vi "Phoenix.vi"(9 "Com UDP":T13={"UDP GrSim TX"=TRUE, "Address:"="", "Port:"=20011}, 10 "RefBox UDP RX":T12={"Local IP:"="192.168.2.61", "Server IP:"="224.5.23.1", "Port"="10003"}, 11 "SSL UDP RX":T12={"Local IP:"="", "Server IP:"="224.5.23.2", "Port"="10020"}) -> ()   [LabVIEW 2024]
uses:
  Vision_class/Old vision/Controls/Estimadores.ctl
  Vision_class/Old vision/Decode SSL and Refree Wrapper Package Folder/SSL Referee Game Status.ctl
  Vision_class/Old vision/Draw Field Folder/DrawTargets.ctl
  Vision_class/Old vision/Controls/SSL Field State.ctl
  Vision_class/Old vision/Controls/SSL Detection Frame.ctl
  Vision_class/Old vision/Controls/SSL Detection Robot.ctl
  <vilib>/Analysis/Matrix/Datatypes/RealMatrix.ctl
  Vision_class/Old vision/Controls/SSL Detection Ball.ctl
  Communication_class/Communication.lvclass
  Controls/ComUDP.ctl
  Controls/ComSerial.ctl
  Controls/ComSOS.ctl
  Controls/PhoenixParameters.ctl
  Play_class/PassReceiver.ctl
  Parameters_class/ChoosePassReceiver.ctl
  Game_class/Navigation/Controls/bangBangControlParameters.ctl
  Game_class/PathPlanning/Path Planning/RRT/RRTParameters.ctl
  Controls/PIDParameters.ctl
  Parameters_class/Project.ctl
  Controls/RobotModelTestState.ctl
  Game_class/VelocityPlanningTest/Controls/testMode.ctl
  Controls/RobotModelReplacementTest.ctl
  Controls/grSimReplacement.ctl
  Communication_class/Paths/grSim Packet Command UDP Test Folder/grSim/grSim RobotReplacement.ctl
  Communication_class/Paths/grSim Packet Command UDP Test Folder/grSim/grSim_BallReplacement.ctl
  Game_class/KickValueTest/KickValuetest.ctl
  Game_class/KickValueTest/KickValue.ctl
  Game_class/KickValueTest/BallValue.ctl
  Game_class/VelocityPlanningTest/Controls/velocityPlanningState.ctl
  Game_class/VelocityPlanningTest/Controls/trajectoryState.ctl
  Controls/Enviroment.ctl
  Team_class/KeeperPlay.ctl
  Team_class/OffensivePlay.ctl
  Referee_class/command_interpreted.ctl
  Robot_class/roles.ctl
  Robot_class/tactics.ctl
  Team_class/DefensivePlay.ctl
  Controls/vision_control.ctl
  Game_class/KickForceTest/Controls/kickForceTestState.ctl
  Game_class/KickForceTest/Controls/KickForceEnum.ctl
  Game_class/Replay/ReplayControls.ctl
  Game_class/ParametersFromFile/ParametersFromFile.ctl
  Robot_class/robotDisplayFeedback.ctl
  Controls/NewParameters.ctl
  Utilities_class/Style.ctl
  Controls/AllyTeam.ctl
  Zone_class/zones.ctl
  Vision_class/Vision.lvclass
  Game_class/Game.lvclass
  Vision_class/Old vision/Controls/SSL_BallModelStraightTwoPhase.ctl
  Game_class/Game.lvclass/Game.ctl
  Referee_class/Referee.lvclass/Referee.ctl
  Team_class/Team.lvclass/Team.ctl
  Robot_class/Robot.lvclass/Robot.ctl
  Game_class/ParametersFromFile/MainGameConfigs.ctl
  Robot_class/Robot.lvclass
  Events_class/Events.lvclass
  RobotFeedback/RobotFeedback.lvclass/RobotFeedback.ctl
  RobotFeedback/Read id.vi
  RobotFeedback/Read dribblerContactToBall.vi
  Game_class/Write RobotsFeedback.vi
  Robot_class/Read id.vi
  Robot_class/Read role.vi
  Robot_class/Read tactic.vi
  Game_class/Read Referee.vi
  Game_class/Read KeeperTeam.vi
  Game_class/Read OffensiveTeam.vi
  Game_class/Read DefensiveTeam.vi
  Team_class/Read RobotRef.vi
  Team_class/Read DefensivePlay.vi
  Team_class/Read OffensivePlay.vi
  Team_class/Read KeeperPlay.vi
  Referee_class/Read command_interpreted.vi
  Game_class/Write TestTeam.vi
  Game_class/Write DefensiveTeam.vi
  Game_class/Read AllyRef.vi
  Team_class/Write RobotRef.vi
  Game_class/Write NavigationTeam.vi
  Game_class/Write EventsRef.vi
  Game_class/Write OffensiveTeam.vi
  Game_class/Write KeeperTeam.vi
  Ally_class/Ally.lvclass
  C:/Users/moise/Documents/GitHub/SSL_AI/Team_class/Team.lvclass
  RobotFeedback/commCAS.vi
  Referee_class/Referee.lvclass
  Playbook_class/Playbook.lvclass
  <vilib>/Analysis/Matrix/NI_Matrix.lvlib
  Utilities_class/Utilities.lvclass
  RobotFeedback/RobotFeedback.lvclass
  Zone_class/Zone.lvclass
panel:
  in  "accel":dbl
  out "topSpeed":dbl=2466.234375
  out "FPS vision":dbl=64.30864933106373
  out "kick":bool
  in  "Enum":T1=enum."Size"
  in  "Boolean":bool
  in  "robotAngles":dbl[](array[numeric])=[30.0, 150.0, 225.0, 315.0] format="%#_13g"
  out "LastOffensivePlays":T2[](array[typedef])=[enum."5RobotsNormalGamePlay", enum."EnemyPossesionAtOurField", enum."5RobotsNormalGamePlay"]
  out "FPS Read UPD by Cam":dbl=235.84891019160068
  out "DefenseAvoidArea":bool
  in  "AttackerAvoidArea":bool
  out "KeeperPlay":T3=enum."KeeperPlay"
  out "OffensivePlay":T2=enum."5RobotsNormalGamePlay"
  out "DefensivePlay":T4=enum."NormalDefensive"
  out "command_interpreted":T5=enum."Force Start"
  out "robotFeedback":cluster{"id":u32, "dribblerContact":bool}[](array[cluster])
  in  "Life Time":dbl=2.5
  in  "timeToValidateBall":dbl=1.0
  in  "Line?":bool
  in  "BallOut":bool
  out "replaceBall":bool
  out "replaceRobots":bool
  out "grSIM replacement":T6
  out "robotControlResponseConnectionID":refnum<k16>
  out "robotControlResponseErrorOut":errorcluster
  out "error out 2":errorcluster={"status"=TRUE, "code"=66, "source"="UDP Read in Phoenix.vi"}
  in  "Debug Ball":bool
  out "NaN?":bool
  out "Log":string
  out "Exit":i32
  in  "Args":string[](array[string])
  out "touch":bool
  in  "Field Size":T9
  in  "Debug":bool=TRUE
  in  "ball velocity máx":dbl=8.0
  in  "ChipKick activated":bool=TRUE
  out "error out":errorcluster
  in  "Draw Graphs":bool
  in  "Test":bool
  in  "Tab Control":T10(tab)=enum."NewParameters"
  in  "ParametersFromFile":T11
  in  "Com Serial":T14={"Serial TX"=TRUE, "Porta:"="COM4"}
  in  "Com SOS":T15={"UDP SOS TX "=FALSE, "SOS Port: 2"=10025, "SOS Port: "=10021, "SOS Address:"="192.168.0.101"}
  out "RefBox RX":bool=TRUE
  in  "Defense\n stretch":i32=2000
  in  "Defense\n width":i32=1000
  in  "Team":enum16{"Azul", "Amarelo"}(ring) caption="Enum"
  in  "Side":enum16{"Esquerdo", "Direito"}(ring) caption="Enum"
  in  "Command":string(combo)="Force Start"
  in  "AttakingOurselves":bool
  out "SSL RX":bool=TRUE
  in  "FIRASim?":bool
  in  "Project":T16
  in  "Envirnoment":T17=enum."realGame"
  in  "ViewState":T18(ring)=enum."Maximized"
  out "RefBox RX 2":bool=TRUE
  out "SSL RX":bool=TRUE
  out "displayFeedbackRobot":T19[](array[typedef]) {"Battery (V)" scale=6.0..8.4}
  out "Side out":enum16{"Esquerdo", "Direito"}(ring) caption="Enum"
  out "Team out":enum16{"Azul", "Amarelo"}(ring) caption="Enum"
  out "Envirnoment out":T17=enum."realGame"
  in  "AI Parameters":T20={"Defensive Marker"=enum."SecondMostDangerous", "TimeoutDistanceInX"=600.0, "TimeoutDistanceInY"=600.0, "DistanceForaStillBall"=0.0, "TouchDistance"=150.0, "AttackerFarback"=1500.0, "MinDistToKick"=400.0, "Type of Marker"=enum."BlockOurGoal", "Type of Defense "=enum."Barreira", "PassAngle"=0.045, "KickRange"=60.0, "KickForce"=34.0, "KickEps"=0.1, "KickAngle"=5.0, "PassForceMult"=1.2, "DistanceToKickingAngle"=150.0, "DistanceToBallOut"=600.0, "DistanceStop"=750.0, "DistanceBehindAttacker"=200.0, "Area"=enum."Square", "DistanceForPossession"=350.0, "DistanceToConsirerRobotArrive"=50.0, "DistanceToGoAroundBall"=60.0, "DistanceInFrontOfAttacker"=200.0, "TimeoutDistanceBetweenRobots"=300.0, "MaxOutputAngle"=3.0, "MaxOutputXY"=3.5, "MaxDeceleration"=1.0, "MaxControlIncrement"=1.0, "MaxAcceleration"=4.5, "AngularToleranceForPossession"=0.3, "MaxVelBallToBeginDuelist"=0.5, "ZigZagAngle"=0.0, "PID gains Vel"={"(Kc)"=0.1, "(Ti, min)"=0.0, "(Td, min)"=2.0}, "Number of Offensive"=enum."Auto", "Shoot Out?"=FALSE, "DefenseAvoidArea"=FALSE, "InvertKick"=[], "Simple Pass"=FALSE, "ShootOutForce"=20.0, "dtPosEstBall"=0.3, "AttkIgnoreBallObst"=2500.0, "BarrierDist"=130.0, "PassReceiver"=enum."Auto", "GoalieInFrontGoal"=120.0, "RollToPass"=FALSE, "PassReceiver"=enum."Auto", "OldRRT"=FALSE, "Dribbler"=FALSE, "VelNearBall"=2.0, "ChipKick Force"=2.5, "ForcePass\nInGame"=10.0, "bangBangParameters"={"MaxVSent"=4.0, "MaxVNorm"=4.0, "MaxVAng"=8.0, "VAngCircle"=3.0, "LBeginCircle"=300.0, "DistToDestOrientation"=300.0, "MaxVAngToTurn"=8.0, "AtkDistToDestOrientation"=3500.0, "KepperMaxVSent"=4.0, "VelNearEnemy"=1.5}, "BallVelToAbortPass"=0.1, "BallVelToFinishPass"=1.0, "minDistanceToPass"=1000.0, "dribbler_rpm"=1.0, "AttackerAngle\nToTurnInDegrees"=5.0, "AttackerAngle\nToShootInDegrees"=0.5, "distToActivateDibbler"=1000.0, "StopVelocity"=1.2, "timeoutToShoot"=10.0, "DistanceArea"=100.0, "MinDistanceEnemy\nToBallToMark"=750.0, "DisableStopAvoidArea"=FALSE, "RRT Parameters"={"threshold"=120.0, "Step"=120.0, "GoalProb"=0.1, "WayPointProb"=0.6}, "PID per ID"=[]} {"RRT Parameters"."WayPointProb" format="%#_13g"; "RRT Parameters"."GoalProb" format="%#_13g"}
  in  "NewParameters":T26={"PenaltyDistance"=1800.0, "DistanceAttackerToBackBall"=40.0, "Division"=enum."Div B", "DistanceToAvoidyEnemyRobot"=600.0, "BallPlacementDistance"=900.0, "DisatanceBehindBallToStealBall"=600.0, "MaxDistanceToPositionKickoff"=2000.0, "BlockEnemyTarget"=TRUE, "MaxStopVAng"=4.0, "DistanceMarkerToEnemy"=600.0, "IgnoreDribblerContact"=FALSE, "DistanceToBeginEnemyPosession"=400.0, "GoToBallWhenEnemyNotMoving"=TRUE, "EnemyDistanceToReduceVelocity"=500.0, "TurnOnEnemyDistanceToReduceVelocity"=TRUE, "EnemyDistanceToShootOutBall"=0.0, "DefenseKickBall"=TRUE, "MoreKickToGoal? (0-0.3)"=0.25, "ChipKickInEnemyField"=TRUE, "ShootOutRobotId"=4.0, "FieldLenghtDenominatorInShootOut"=-18.0, "AdjustPositionInBallPlacement"=FALSE, "PowerGodPass"=0.75, "VelocityAbortEnemyPos"=3.0, "MaxDistToBeginPass"=300.0, "MinDistToBeginPass"=150.0, "VelocityInDirects"=0.3, "BadDribblerIDs"=[], "NewKickToDistanceAroundBall"=300.0, "PowerAvoidColisionMarker"=1.0, "DistanceToAvoidColisionMarker"=0.0, "AvoidBallKick"=70.0, "DistanceTryKick"=-250.0, "SuicideKickDIstance"=80.0, "AdjustFirstKickDistance"=100.0, "AvoidAimLessKick"=0.7, "DistanceToAvoidyEnemyShootRobot "=100.0, "NumberOfMarkers"=1.0, "PotField"=FALSE, "PIDLateral"=TRUE, "MinDistanceFirstKickX"=100.0, "MinDistanceFirstKickY"=750.0, "FractionOfDistToTouchGround\nAfterChipKick"=0.7, "FractionOfKickxWhen\nComposedWithKickz"=0.7, "Style"=enum."Offensive", "MoveInTurnState"=TRUE, "DistFromEnemyToConsider\nMoveInTurnState"=400.0, "CascadePID"=TRUE, "TurnAroundParameters"={"Radius"=270.0, "Multiplier"=2.0, "ChordAngle"=100.0}, "SafeDriveVel"=0.2, "DistanceToGoToBackBall"=500.0, "minDistanceToNotFinish\nEnemyPossession"=100.0, "OneTouchShot"={"angleFactor"=1.0, "maxAngle"=70.0, "Attack"=TRUE, "Defense"=TRUE}, "OpenAngleToGoal"={"minAngle"=2.0, "maxAngle"=15.0, "minEvaluation"=0.5}, "ShotInterception"={"shotSpeed"=6.0, "minEnemySpeed"=0.7, "maxEnemySpeed"=2.5, "minEvaluation"=0.5}, "AllyTeamArray"=[enum."Defender", enum."Defender", enum."Keeper", enum."Attacker", enum."Attacker", enum."Attacker"], "maxDefendersNumber"=2, "Zone"={"GuardPositionArray"=[[1000.0, 0.0], [1000.0, 1500.0], [1000.0, -1500.0], [875.0, 0.0], [3125.0, 1750.0], [3125.0, -1750.0], [875.0, 1500.0], [875.0, -1500.0], [3125.0, 1750.0], [2625.0, 0.0], [3125.0, -1750.0]], "ZoneMidField"=[1750.0, 0.0], "CenterForwardWidth"=2000.0}, "MinEvaluationToShoot"=0.3, "PassInterception"={"maxPassSpeed"=6.0, "minPassSpeed"=3.0, "minEnemySpeed"=0.7, "chipPassDistance"=1000.0, "chipPassEvaluation"=0.7, "minEvaluation"=0.5, "maxEnemySpeed"=2.5}, "PassDistance"={"maxDistance"=3000.0, "minDistance"=1500.0}, "receiverSpeed"=3.0, "maxBallSpeed"=6.0, "slackTime"=0.1, "Turning radius"=250.0, "Turning v_ang"=2.0, "AlignError"={"Distance"=60.0, "Orientation"=15.0, "V_norm(m/s)"=0.15, "V_ang (rad/s)"=0.15}, "RobotRadius"=85.0, "KickerDistance"=75.0, "keeper angle  to cover goalpost"=60.0, "a_slide"=-1.0, "a_roll"=-1.0, "k_switch"=0.99, "Penalty"=0} {"Penalty" items=["Default", "DirectKick", "IndirectKick"]}
  in  "Goalie":string(combo)="2"
  in  "ReplayControls":T29={"Slide"=0.0, "Enable"=FALSE, "FPS"=300.0, "On"=FALSE, "Play"=FALSE, "CopyFile"=FALSE, "CopyFilePathRelativeToLogFolder"="teste1.txt", "ReadFromFile"=FALSE, "ReadPathRelativeToLogFolder"="teste1.txt", "FrameBufferSize"=100000.0, "Speed"=1.0} {"Slide" scale=0.0..10.0}
  out "Slide out":dbl(slide) scale=0.0..10.0
  out "Keeper Team":cluster{"id":i32, "role":T30, "tactic":T31}[](array[cluster])=[{"id"=2, "role"=enum."KeeperRole", "tactic"=enum."DefendGoal"}]
  out "Offensive Team":cluster{"id":i32, "role":T30, "tactic":T31}[](array[cluster])=[{"id"=3, "role"=enum."Shoot", "tactic"=enum."Shoot"}]
  out "Defensive Team":cluster{"id":i32, "role":T30, "tactic":T31}[](array[cluster])=[{"id"=1, "role"=enum."DefenderArea", "tactic"=enum."DefendGoal"}, {"id"=0, "role"=enum."DefenderArea", "tactic"=enum."DefendGoal"}]
  in  "TestMode IDS":dbl[](array[numeric])
  out "SSL Referee Game Status":T32={"Stage"="Post Game", "Command"="Force Start", "Time Left"=0.0, "Yellow Team"="RoboIME", "Blue Team"="Warthog Robotics", "Yellow Score"=0, "Blue Score"=5, "Yellow Red Cards"=0, "Blue Red Cards"=0, "Yellow Yellow Cards"=3, "Blue Yellow Cards"=0, "Yellow Timeouts Left"=2, "Blue Timeouts Left"=2, "Yellow Timeout Remaining"=150.0, "Blue Timeout Remaining"=150.0, "Yellow Goalie Id"=3, "Blue Goalie Id"=6, "Time"=timestamp(3779822234.55011 s since 1904-01-01), "Point"={"x"=0.0, "y"=0.0}} {"Time" format="%<%.3X %x>T"; "Blue Timeout Remaining" format="%<%M:%S>t"; "Yellow Timeout Remaining" format="%<%M:%S>t"; "Time Left" format="%<%M:%S>t"}
  out "FPS SetParameters":dbl=4.988732988868486
  out "FPS Defensive":dbl=81.16887087847226
  out "FPS Com":dbl=68.21282028346764
  out "FPS Draw Field":dbl=28.457509856616845
  out "FPS Graph":dbl=22.05084954808498
  out "FPS referee":dbl=38.86515306793774
  out "FPS Events":dbl=60.02408230917689
  in  "zigzag Points":cluster{"x":dbl, "y":dbl, "Angle":dbl}[](array[cluster])=[{"x"=-500.0, "y"=-500.0, "Angle"=0.0}, {"x"=-500.0, "y"=500.0, "Angle"=0.0}, {"x"=500.0, "y"=500.0, "Angle"=0.0}, {"x"=-500.0, "y"=500.0, "Angle"=0.0}]
  in  "TestMode":bool
  in  "Tests":enum16{"zigzag", "goto"}(ring)
  in  "Offensive ids":dbl[](array[numeric])
  in  "Defensive ids":dbl[](array[numeric])
  out "FPS Read UDP":dbl=235.84891019160068
  out "FPS getCam":dbl=81.16887087847226
  out "FPS grSimTest":dbl=0.9997000878761829
  out "FPS RobotFeedback":dbl=414.95798286072704
  in  "feedbackId":u32=5
  out "FPS Debug":dbl=57.53789145633843
  out "FPS ViewState":dbl=0.9997000878761829
  out "FPS ReplaceErForce":dbl=69.54111166856396
  out "FPS Replay":dbl=305.79777980947716
  out "FPS Offensive":dbl=81.16887087847226
  out "FPS Navigation":dbl=96.15270345115962
  out "FPS RRTOffensive":dbl=81.16887087847226
  out "FPS Keeper":dbl=81.16887087847226
  in  "RobotModelFolder\nFrom RobotModel":string
  in  "grSimTest":bool
  out "RobotModelState":T33 {"progress" scale=0.0..100.0}
  in  "Test":T34=enum."TurnTest"
  in  "Reaplacement Tests":T35={"grSIM replacement"={"robots"=[], "ball"={"x"=0.0, "y"=0.0, "vx"=0.0, "vy"=0.0}}, "replace active"=FALSE, "TestParameters"={"Start"=FALSE, "V_sent(not used\nmore)"=0.0, "id"=1, "Samples"=0.0, "V_sample"=0.0, "delta"=0.2, "Test number"=0.0}, "Dest_array"=[[{"dest_x"=0.0, "dest_y"=0.0, "dest_orientation"=90.0, "dest_vel"=0.0}, {"dest_x"=-1500.0, "dest_y"=-1000.0, "dest_orientation"=90.0, "dest_vel"=0.0}]], "replaceBall"=FALSE, "ballVelocity"=0.0, "timeoutKick"=0.0, "KickValueTest"={"ForceValue"={"delta_kick"=10.0, "kick_min"=40.0, "kick_max"=70.0}, "BallValue"={"delta_ball"=1.0, "v_min_ball"=-5.0, "v_max_ball"=2.0}, "Samples"=10.0, "Start"=FALSE, "id"=0, "RobotStopKick"=FALSE}, "StateSpaceTestParameters"={"Start"=FALSE, "uMaxPos"=0.4, "frequency"=40, "Samples"=5000.0, "uMinPos"=-0.4, "holdingFrequency"=50.0, "uMaxAngle"=1.5, "uMinAngle"=-1.5, "id"=0.0}}
  out "velocityPlanningState":T39
  out "kickForceTestState":T41
  in  "ABORT!!!!!!!!!":bool
  in  "Id camera\ninf dir":dbl=2.0
  in  "Id camera\ninf esq":dbl
  in  "Id camera\nsup dir":dbl=3.0
  in  "Id camera\nsup esq":dbl=1.0
  in  "ignore left?":bool
  in  "ignore rigth?":bool
  in  "Estimador":T43
  in  "Draw Targets?":T44={"Attacker"=TRUE, "Striker"=TRUE, "Goalie"=TRUE, "Defender"=TRUE, "kick"=TRUE, "Est Ball"=TRUE, "Est Robot"=FALSE, "Path S"=FALSE, "Path C"=FALSE, "Dngr.Enemy"=TRUE, "2nd Striker"=TRUE}
  in  "Draw Field":bool=TRUE
  in  "id 3":dbl
  in  "id 2":dbl
  in  "id 1":dbl
  out "Robot":cluster{"Modulo":dbl, "Modulo":dbl}(graph)
  out "Robot":cluster{"Modulo":dbl, "Modulo":dbl}(graph)
  out "Ball_z":cluster{dbl}(graph)
  out "Ball_vel":cluster{"Modulo":dbl}(graph)={"Modulo"=0.00013064281513160085}
  out "Robot 2":cluster{"Modulo":dbl, "Modulo":dbl}(graph)
  out "Intensity Graph":dbl[][](graph)=[[0.6439849956797391, 0.6468713754975447, 0.6496267341345192, 0.652238572304966, 0.6546945914065111, 0.6569828206385522, 0.6590917480472425, 0.6610104531776768, 0.6627287387777703, 0.6642372588298054, 0.6655276400974819, 0.6665925943802322, 0.6674260187684942, 0.6680230813965182, 0.6683802904894185, 0.6684955448902967, 0.6683681647181078, 0.6679989013283556, 0.6673899263063497, 0.6665447997918109, 0.6654684189894605, 0.6641669482401004, 0.6626477324874634, 0.6609191963614056, 0.6589907313934924, 0.6568725740785315, 0.6545756775930542, 0.6521115799803755, 0.6494922715198369, 0.6467300638252331], [0.5222937405333601, 0.5231869629637252, 0.5239943362540308, 0.5247101824413543, 0.52532911767851, 0.5258461241958458, 0.5262566213380001, 0.5265565340667843, 0.5267423572653613, 0.5268112141815539, 0.0, 0.0, 0.0, 0.0, 0.0, 0.0, 0.0, 0.0, 0.0, 0.0, 0.0, 0.5287814171255, 0.5286937870670604, 0.5284874875448279, 0.528165514466294, 0.5277314971463923, 0.5271896382619184, 0.5265446479979172, 0.5258016740780306, 0.5249662293687821], [0.5243108011349319, 0.5252727330245326, 0.5261444870226399, 0.5269197571460855, 0.5275925456518729, 0.5281572456923016, 0.5286087233355957, 0.5289423970418683, 0.5291543126011065, 0.5292412115270873, 0.0, 0.0, 0.0, 0.0, 0.0, 0.0, 0.0, 0.0, 0.0, 0.0, 0.0, 0.5312555283014799, 0.531148541258167, 0.5309147334258806, 0.5305574960630276, 0.5300809214217669, 0.5294897325094089, 0.528789206378234, 0.5279850929840529, 0.5270835316357332], [0.5264005985006444, 0.5274375464102949, 0.5283797700154165, 0.5292202549028815, 0.5299523078652293, 0.5305696520068088, 0.5310665216503045, 0.5314377547718625, 0.5316788805718677, 0.5317861997540423, 0.0, 0.0, 0.0, 0.0, 0.0, 0.0, 0.0, 0.0, 0.0, 0.0, 0.0, 0.5338465727897175, 0.533717726205971, 0.5334531606291533, 0.5330567236191915, 0.5325330397061038, 0.5318874279831642, 0.5311258125056296, 0.5302546279631231, 0.5292807230507116], [0.5285662503328791, 0.5296852053449023, 0.5307046714576859, 0.5316168338771309, 0.5324142100725614, 0.5330897594010063, 0.5336369931617511, 0.5340500823751366, 0.5343239604059156, 0.534454417485094, 0.0, 0.0, 0.0, 0.0, 0.0, 0.0, 0.0, 0.0, 0.0, 0.0, 0.0, 0.5365629139453422, 0.5364093510158129, 0.5361103387816856, 0.5356702529426275, 0.5350943316805415, 0.534388578678175, 0.5335596581660944, 0.5326147849917315, 0.5315616126264067], [0.530810941515476, 0.5320196640742294, 0.5331239182202973, 0.5341149834981508, 0.5349844798656975, 0.5357244942687414, 0.5363277085379299, 0.5367875253810392, 0.5370981889968558, 0.5372548967238185, 0.0, 0.0, 0.0, 0.0, 0.0, 0.0, 0.0, 0.0, 0.0, 0.0, 0.0, 0.5394137186527801, 0.5392321704552452, 0.5388945137568703, 0.538405737348643, 0.5377717888550684, 0.5369994602365521, 0.5360962644990299, 0.5350703072530617, 0.5339301566368765], [0.5, 0.5, 0.0, 0.5, 0.5, 0.5066529272415466, 0.517019262787706, 0.5275201684492046, 0.5297293327425996, 0.5316111368002591, 0.5333710118128144, 0.5349985550707285, 0.5364840988483267, 0.5378188684801058, 0.538995128931668, 0.5400063152202025, 0.5408471424402213, 0.5415136917739422, 0.5420034696827905, 0.5423154384459877, 0.5424500172754717, 0.5424090543338507, 0.5421957710458796, 0.541814681064705, 0.5412714870776745, 0.5405729592739007, 0.5397267997209609, 0.5387414971037089, 0.5376261762704322, 0.5363904468306431], [0.5, 0.0, 0.5, 0.5, 0.5, 0.5057980548256944, 0.5167190676488145, 0.5277984573316296, 0.5321180249791597, 0.5341264059593971, 0.536005140664426, 0.5377425503661245, 0.5393277633139989, 0.540750901205234, 0.5420032526340018, 0.5430774277559435, 0.5439674888781911, 0.5446690524505748, 0.5451793589542318, 0.5454973084034875, 0.5456234605210856, 0.5455600000336607, 0.5453106688753424, 0.5448806683029468, 0.5442765349461464, 0.5435059955890522, 0.5425778059759003, 0.5415015791440235, 0.5402876087253506, 0.5389466923533661], [0.5, 0.0, 0.5, 0.5, 0.5, 0.504715272768115, 0.5162326422208229, 0.5279362595825823, 0.5346060791426129, 0.5367531166676786, 0.5387622106817106, 0.5406202140215307, 0.5423148652447439, 0.5438350094357985, 0.5451708043141312, 0.5463139044557284, 0.5472576169992699, 0.5479970231504517, 0.5485290610791688, 0.5488525673479827, 0.5489682757200838, 0.5488787739581055, 0.548588420926096, 0.5481032278368505, 0.547430708754809, 0.5465797064046768, 0.5455601999104328, 0.5443831012921669, 0.543060047401502, 0.5416031935237681], [0.5, 0.5, 0.5, 0.5, 0.5, 0.5033702971299159, 0.5155294540754811, 0.5279075577842101, 0.5371988044640221, 0.5394980618556215, 0.5416504589871762, 0.5436411534507292, 0.5454562742371086, 0.5470831842407143, 0.5485107262381271, 0.549729443327636, 0.5507317654747785, 0.5515121549736335, 0.5520672052495649, 0.5523956893963521, 0.5524985570286525, 0.5523788802880293, 0.5520417520106231, 0.5514941410014329, 0.5507447109432875, 0.5498036106118204, 0.548682243727346, 0.5473930269473528, 0.5459491442256365, 0.5443643051016093], [0.5, 0.0, 0.5, 0.5, 0.5, 0.501723337807691, 0.5145737969094563, 0.5276816527452828, 0.539901738020814, 0.5423684840545748, 0.544678795064896, 0.5468158651059939, 0.548763952179681, 0.5505086916039632, 0.5520373909065077, 0.5533392948812512, 0.5544058102137159, 0.5552306805251843, 0.5558101047351675, 0.5561427941650955, 0.5562299666256902, 0.5560752786398862, 0.5556846997399082, 0.5550663352431152, 0.5542302058955322, 0.5531879941638177, 0.5519527677024318, 0.5505386906291886, 0.5489607327663306, 0.5472343860438509], [0.5, 0.5, 0.5, 0.0, 0.5, 0.5, 0.513323810149363, 0.5272222292967464, 0.5413555034171351, 0.545372089252212, 0.5478568552825293, 0.5501558299140171, 0.5522510880532872, 0.5541262432053284, 0.5557668026874419, 0.5571604879577896, 0.5582975065397346, 0.5591707638189193, 0.5597760056055529, 0.5601118856126258, 0.560179955661175, 0.5599845802010454, 0.5595327803390917, 0.558834015725048, 0.5578999151435897, 0.5567439683533887, 0.5553811925405516, 0.5538277867347433, 0.5521007867625445, 0.5502177319289627], [0.5030290120210578, 0.5, 0.5, 0.5, 0.5, 0.0, 0.5117302905492986, 0.5264862123520307, 0.5415236106039867, 0.5485170534319759, 0.5511950586376688, 0.5536736189241434, 0.5559322518850847, 0.5579521947210897, 0.559716834239406, 0.5612120960573637, 0.5624267756439888, 0.5633527960732316, 0.5639853807195848, 0.5643231333658303, 0.5643680229802749, 0.564125275363959, 0.5636031785606127, 0.5628128129936374, 0.5617677204510374, 0.5604835280939083, 0.5589775445488349, 0.5572683449063265, 0.5553753602292995, 0.5533184851915023], [0.5096738533141254, 0.5, 0.0, 0.5, 0.5, 0.0, 0.5097352472054201, 0.5254223606922725, 0.5414467741804555, 0.5518120180822061, 0.5547046620267404, 0.5573830097164709, 0.5598235707413324, 0.5620047767833217, 0.5639075048575061, 0.5655155528726792, 0.5668160450496404, 0.5677997475315492, 0.5684612788578935, 0.5687992055308398, 0.568816019216649, 0.568517998645437, 0.5679149654307455, 0.5670199483119681, 0.5658487743273963, 0.5644196079102766, 0.5627524597938817, 0.5608686870066167, 0.5587905033595993, 0.5565405169912374], [0.516955790733465, 0.5066285557747776, 0.5, 0.0, 0.5, 0.5, 0.5072701392875174, 0.5239695314983943, 0.541073264832635, 0.5552660694981667, 0.5583978123898882, 0.5612991138027281, 0.563942930021289, 0.5663043648081226, 0.5683613095775818, 0.5700950279399516, 0.571490655348212, 0.572537588077354, 0.5732297414054055, 0.5735656642102906, 0.5735485055962134, 0.5731858378391785, 0.5724893480888296, 0.5714744181612061, 0.5701596168558425, 0.5685661322146024, 0.5667171719463916, 0.5646373590387596, 0.5623521467180385, 0.5598872728680279], [0.5249487634715576, 0.5141904050979103, 0.5025947575551912, 0.5, 0.5, 0.5, 0.5042537205940862, 0.5220545299700755, 0.540340447967038, 0.5588886946692861, 0.562287591713188, 0.565438514703838, 0.5455419855800085, 0.5, 0.5, 0.5342879082031676, 0.5764793487533976, 0.5775957928482389, 0.5783203022731214, 0.5786514378008085, 0.5785931789907278, 0.5781546957475185, 0.5773499565184732, 0.5761971991198592, 0.574718296693452, 0.5729380548400017, 0.5708834765191856, 0.5685830291445819, 0.5660659439863411, 0.5633615722146391], [0.5337363644702983, 0.5225400834328151, 0.510401523388834, 0.5, 0.5, 0.5, 0.5005893960889117, 0.5195894341741296, 0.5391722095775875, 0.5592078343908193, 0.5663880488793314, 0.5698194154784916, 0.0, 0.0, 0.0, 0.0, 0.0, 0.0, 0.0, 0.5840893878260711, 0.5839813775329774, 0.5834537145121796, 0.5825231724811675, 0.5812114737361801, 0.5795444925607558, 0.5775513805416406, 0.5752636614777369, 0.572714339885015, 0.5699370606227345, 0.5669653489221246], [0.5434130880523297, 0.5317772723107352, 0.5190791767339176, 0.5053274416629292, 0.5, 0.5, 0.5, 0.5164682539233363, 0.5374756944628968, 0.5590393816647918, 0.5707142094670336, 0.0, 0.0, 0.0, 0.0, 0.0, 0.0, 0.0, 0.0, 0.0, 0.589748684614559, 0.5891157745514678, 0.5880385063652243, 0.5865428769355601, 0.5846596292330895, 0.5824231579734724, 0.57987039047604, 0.5770396991132887, 0.5739698920465579, 0.5706993171818038], [0.5540856772245775, 0.5420159070475646, 0.5287466765364334, 0.5142786522168231, 0.5, 0.5, 0.5, 0.5125627419727183, 0.5351371511369011, 0.5583954659909859, 0.0, 0.0, 0.0, 0.0, 0.0, 0.0, 0.0, 0.0, 0.0, 0.0, 0.0, 0.5951780824377859, 0.5939290278138185, 0.5922197606755157, 0.5900869786217304, 0.5875714291248739, 0.5847165198753287, 0.5815669885778579, 0.5781676901151251, 0.5745625422087477], [0.5658745397125027, 0.5533862088673918, 0.5395416737610884, 0.5243302615366188, 0.5077678627448103, 0.5, 0.5, 0.5077171236885265, 0.5320166103287423, 0.0, 0.0, 0.0, 0.0, 0.0, 0.0, 0.0, 0.0, 0.0, 0.0, 0.0, 0.0, 0.0, 0.6002318556534632, 0.5982734715535951, 0.5958517314606255, 0.5930151138022934, 0.5898148237318674, 0.5863031625241878, 0.5825320704268889, 0.578551890410509], [0.5757188625631271, 0.5660369018278409, 0.5516235674758034, 0.5356486525004553, 0.5181162829360846, 0.5, 0.5, 0.5017414448498555, 0.0, 0.0, 0.0, 0.0, 0.0, 0.0, 0.0, 0.0, 0.0, 0.0, 0.0, 0.0, 0.0, 0.0, 0.6069887113999217, 0.6047386312321031, 0.601981017615009, 0.5987737986810805, 0.5951775913993492, 0.5912536994650027, 0.5870623650075526, 0.5826613270852558], [0.5794487643784063, 0.5801375574435398, 0.5651769584236707, 0.548429343018279, 0.5298813849620045, 0.5095626676546583, 0.5, 0.5, 0.0, 0.0, 0.0, 0.0, 0.0, 0.0, 0.0, 0.0, 0.0, 0.0, 0.0, 0.0, 0.0, 0.0, 0.0, 0.6116534018502551, 0.6085038419425388, 0.6048673876157777, 0.6008160493416987, 0.5964218582710867, 0.5917547748069166, 0.5868810219428972], [0.5832247124850207, 0.5886428272318525, 0.5804154637355169, 0.5629023501824675, 0.5433029747011735, 0.5216290423665696, 0.5, 0.5, 0.0, 0.0, 0.0, 0.0, 0.0, 0.0, 0.0, 0.0, 0.0, 0.0, 0.0, 0.0, 0.0, 0.0, 0.0, 0.6190597064656443, 0.6154508862457304, 0.6113155516933337, 0.6067395409248063, 0.601807673948094, 0.5966012637190645, 0.5805886292963331], [0.5870207335052878, 0.5930044558218424, 0.5975857813886192, 0.579338364539929, 0.5586682461739926, 0.5355591341181114, 0.5100676917648723, 0.5, 0.0, 0.0, 0.0, 0.0, 0.0, 0.0, 0.0, 0.0, 0.0, 0.0, 0.0, 0.0, 0.0, 0.0, 0.0, 0.6270033555281816, 0.6228541035915198, 0.6181368916955089, 0.6129543736721348, 0.6074066078885175, 0.6015881201427595, 0.5712310912947379], [0.5908026291177239, 0.597415988597139, 0.6039499851783565, 0.5980556757627397, 0.5763217457407289, 0.5517111488900057, 0.5242524791598275, 0.5, 0.0, 0.0, 0.0, 0.0, 0.0, 0.0, 0.0, 0.0, 0.0, 0.0, 0.0, 0.0, 0.0, 0.0, 0.0, 0.6355340005590409, 0.6307459953213602, 0.6253476890411316, 0.6194622105488748, 0.6132077408891132, 0.5944485700779896, 0.559508657573544], [0.5945259631909249, 0.6018389313417347, 0.6091164837361313, 0.6162621379890453, 0.5966771102877683, 0.57052445042188, 0.5409509926850754, 0.5080702811186034, 0.0, 0.0, 0.0, 0.0, 0.0, 0.0, 0.0, 0.0, 0.0, 0.0, 0.0, 0.0, 0.0, 0.0, 0.0, 0.6447047894767861, 0.6391584077521367, 0.6329600695161235, 0.626257837560904, 0.6191913637076513, 0.5824151369126421, 0.5449314798925682], [0.5981336394832157, 0.6062217631644599, 0.6143338667475075, 0.6223636051275623, 0.6202304924223678, 0.5925394005667843, 0.5607218836482615, 0.524845896149073, 0.0, 0.0, 0.0, 0.0, 0.0, 0.0, 0.0, 0.0, 0.0, 0.0, 0.0, 0.0, 0.0, 0.0, 0.6601467793219282, 0.6545715247434784, 0.6481206064622234, 0.6409793311891968, 0.6333260811314694, 0.6108901914763214, 0.5670217150595808, 0.5283909036288752], [0.6015530293280853, 0.6104965104556885, 0.6195428514626099, 0.6285764995346007, 0.637455586696884, 0.6184214444158891, 0.5842719514542074, 0.5451097412994319, 0.5011777035477128, 0.0, 0.0, 0.0, 0.0, 0.0, 0.0, 0.0, 0.0, 0.0, 0.0, 0.0, 0.0, 0.0, 0.6717760699199902, 0.6651910104681699, 0.6576562688255065, 0.6494000859863929, 0.6406375720723887, 0.5948917546399709, 0.5474882314759214, 0.5267186795633867], [0.604692633827302, 0.6145745906553617, 0.6246625974142697, 0.6348336464758179, 0.6449309477031051, 0.6489893586165244, 0.6124992527434667, 0.5697803198992892, 0.5209992821071739, 0.5, 0.0, 0.0, 0.0, 0.0, 0.0, 0.0, 0.0, 0.0, 0.0, 0.0, 0.0, 0.6909428739567487, 0.6844364790787618, 0.676618093782485, 0.6677788622901877, 0.6582007236957254, 0.6306482962190141, 0.5738896789021376, 0.5342021706161623, 0.5243704942800553], [0.6074383138912121, 0.6183418699492648, 0.6295845892887767, 0.6410394297386267, 0.6525365640804731, 0.6638592427128922, 0.6465475783985548, 0.600069354215026, 0.5458130566242012, 0.5, 0.525314095582295, 0.0, 0.0, 0.0, 0.0, 0.0, 0.0, 0.0, 0.0, 0.0, 0.7066737054793406, 0.7061169120444784, 0.6982346511592952, 0.6889006215027086, 0.6784846218434247, 0.6673355169369155, 0.6084363372128936, 0.5465601720516025, 0.531609261387349, 0.5212261638975573], [0.6096492064184444, 0.6216529510928035, 0.634165164874749, 0.6470606289786731, 0.6601608801553158, 0.6732262474564079, 0.6859509276430754, 0.6375866925714034, 0.5772310101720589, 0.5072493179037366, 0.499540937704119, 0.546067286163326, 0.5407678436542607, 0.4337619972764159, 0.0, 0.0, 0.0, 0.4380369343909474, 0.5905636251332165, 0.6647533030114673, 0.7057031148726275, 0.7228943630556781, 0.7132791651432348, 0.702071086911038, 0.6897419720210722, 0.6546970744892191, 0.5782955302699693, 0.5399568862330024, 0.5280539673243523, 0.5171506202243129], [0.6111535819232568, 0.6243248444346243, 0.6382166427433608, 0.6527148676718605, 0.6676406942024108, 0.6827369338963128, 0.6976569509098829, 0.6844805396602299, 0.6175102251133894, 0.5347815534498871, 0.47527105414674986, 0.5258884410168275, 0.509929656844837, 0.40654026256984704, 0.36688717497785717, 0.3729981123371375, 0.37735566199155346, 0.4026367138737522, 0.5770663626678668, 0.6611640085664815, 0.7070417530256258, 0.7322315636622739, 0.7296720228305553, 0.7161330450999163, 0.7014757171951645, 0.6219867542975964, 0.5496878700761858, 0.5359053230738547, 0.5233601260061715, 0.5294373304269239], [0.6117451059767227, 0.6261304104145115, 0.6414972261113513, 0.6577564500368268, 0.6747428703061993, 0.6921934712996258, 0.709726644610952, 0.7268271616342659, 0.6698505894264419, 0.5649018194179795, 0.0, 0.5026104012498976, 0.5110083733294487, 0.38198318878852316, 0.377739989735005, 0.38511219478098113, 0.39031605964008875, 0.3930992958028493, 0.5659358455924772, 0.6602393080963911, 0.7108856048052159, 0.7379491146999664, 0.7332096282067008, 0.7169022609280854, 0.6727076269376518, 0.5685364203195044, 0.5416090019579305, 0.5304414324632617, 0.5338856793821974, 0.579555252358676], [0.61118025938241, 0.6252486868244983, 0.6408841231911117, 0.6588437475127784, 0.6792768844593, 0.7012968635039972, 0.7145854378145409, 0.7273563395017584, 0.7164700934021416, 0.6088502547870566, 0.4694971139156848, 0.4734220109518266, 0.5177195471990297, 0.3789291615775281, 0.3901207083940296, 0.3991545679397008, 0.40546617232507265, 0.40869359476243877, 0.5573295745194661, 0.6622611399727947, 0.7174712474594367, 0.7385374303946401, 0.7201930235639199, 0.7038009966062881, 0.599931360505176, 0.5329535704166134, 0.5221025033151845, 0.5315250905493286, 0.5954808817640701, 0.6291097280836353], [0.5973921980704098, 0.6102648251187587, 0.6255361818786611, 0.6436827766158082, 0.6651119103879447, 0.6900203508387239, 0.7081212781386476, 0.7198083753975697, 0.7295065081854478, 0.6518728941031504, 0.5292881847355817, 0.4333107858288658, 0.5052862440387922, 0.37553682715059666, 0.4043402957507283, 0.41561332006666946, 0.4234095651637181, 0.42719320499817015, 0.5515083819974024, 0.6676148335341843, 0.7270770949948867, 0.7148312712287904, 0.6960895537440699, 0.6434398549714954, 0.516353633824487, 0.5068207117835309, 0.5078974582878288, 0.5965487582463901, 0.6426238343469461, 0.628170025222976], [0.5795576624161642, 0.5909041346678255, 0.6048841444201841, 0.6223095673050649, 0.6440228420650154, 0.6706707259907424, 0.698608616975367, 0.7080536616091698, 0.7135951501541784, 0.7073710215344642, 0.5716632013548233, 0.4349551394448568, 0.48994265661502945, 0.36875362213937446, 0.42077991478214344, 0.4351504433421148, 0.4449928345573058, 0.44948385599734053, 0.5488738985721191, 0.676815270477588, 0.6970544880300159, 0.6693195130113251, 0.653432715707617, 0.5170003552714878, 0.47903986689402467, 0.4755108364582746, 0.5861386232897302, 0.6342226105684566, 0.6303722053665552, 0.6242711230083491], [0.5577611920723957, 0.566374461979614, 0.5775989167713232, 0.5927215951363398, 0.613315482094443, 0.6408784882788887, 0.6762463949143813, 0.6918453240949315, 0.6900002376537757, 0.6776562416483051, 0.5594766064538007, 0.47557131822592336, 0.46558639370569965, 0.4051035795003807, 0.4398937740444183, 0.458682585267363, 0.47144079794133964, 0.4768465484296066, 0.5500252588829256, 0.673374120504465, 0.6134522983452871, 0.5812630642113112, 0.5271970547011695, 0.4252297706413062, 0.428724357772862, 0.565708412112892, 0.6163223571676623, 0.6182473511302703, 0.6152582273755618, 0.6097653861258364], [0.5317390885834746, 0.5359389806917441, 0.5421397109796083, 0.5522303719708395, 0.5690094135748411, 0.5956536376775549, 0.634440625426208, 0.6775454002462291, 0.6592349831666332, 0.6229197602697047, 0.5541692014705959, 0.32830796115129307, 0.3385647697471023, 0.4681871802462671, 0.46218370817720245, 0.4875070786736397, 0.5, 0.5, 0.5481430327389234, 0.550839062359213, 0.4739241124601594, 0.4507524837027733, 0.3065722382223691, 0.315168726646927, 0.5199095163066917, 0.5790017108007852, 0.5942809223579396, 0.5983759325261079, 0.5967686182075428, 0.5923250042232229], [0.5046350347180243, 0.49915836926361695, 0.49691136295539784, 0.49723115397793555, 0.5049075271101727, 0.5267014540024646, 0.56824875041589, 0.6303248732888446, 0.6340034628468634, 0.5556122961200253, 0.4958275176826772, 0.39897093764181585, 0.40587177354905435, 0.5, 0.4720415530447638, 0.5, 0.5, 0.5, 0.5181303694006516, 0.5, 0.49872243866466043, 0.3663893183077348, 0.25, 0.40221590024966664, 0.4969912299075683, 0.545986132700301, 0.5667257467621772, 0.5739215297834386, 0.5744095763048856, 0.5716014149704008], [0.474395649928083, 0.4566104566709152, 0.4408164154491226, 0.42307419300865884, 0.41056375680629076, 0.41849541133113294, 0.4620094454518258, 0.5420332532004898, 0.6117804243637441, 0.5122512378477078, 0.5, 0.5, 0.5, 0.5, 0.5, 0.5, 0.5, 0.5, 0.5, 0.5, 0.5, 0.25, 0.4424321444023299, 0.4077958718332251, 0.44054917910910885, 0.5046859221117924, 0.5327542606344862, 0.5442718195068214, 0.5477739429488024, 0.5473332789268122], [0.4401519405753111, 0.41516297234994476, 0.37484432715360927, 0.32501637146529516, 0.3232677599129715, 0.3435437212900051, 0.36906544556773924, 0.40394517936877883, 0.5552245153734997, 0.49160429310802084, 0.0, 0.0, 0.0, 0.0, 0.0, 0.0, 0.0, 0.0, 0.0, 0.0, 0.0, 0.4926110914989349, 0.44255977605761665, 0.4019819302442357, 0.3699999923739984, 0.4539897126774899, 0.4916868542287166, 0.5090162526446689, 0.5166312516485162, 0.5194093633162415], [0.3802790470868821, 0.33831516004815787, 0.28806747565163104, 0.29341168833130876, 0.3085024683197401, 0.3279154479695361, 0.3532828467041403, 0.3869152496244338, 0.43608127088439647, 0.49221227693838393, 0.0, 0.0, 0.0, 0.0, 0.0, 0.0, 0.0, 0.0, 0.0, 0.0, 0.0, 0.49222074318511944, 0.4320875750503791, 0.38716946695141297, 0.35362117572960006, 0.39342941273763665, 0.44331849740052126, 0.46810690711997116, 0.48103105143488895, 0.4879346645500562], [0.3562476625898732, 0.3044903974901131, 0.25, 0.0, 0.0, 0.3060217317935241, 0.32881950223441564, 0.3605039518803446, 0.40581752310820857, 0.4723223203348793, 0.0, 0.0, 0.0, 0.0, 0.0, 0.0, 0.0, 0.0, 0.0, 0.0, 0.0, 0.4712378310226052, 0.4053445322961731, 0.36039051365395447, 0.32890447631888836, 0.3236918341765767, 0.3882016398535213, 0.4220209518971517, 0.44139696886561186, 0.45328463816873993], [0.3278516228062476, 0.2628624768609401, 0.25, 0.2562963469883195, 0.26550079876406096, 0.27789853132301096, 0.29514106229803955, 0.32007574227658964, 0.35790319976179363, 0.418737703694432, 0.0, 0.0, 0.0, 0.0, 0.0, 0.0, 0.0, 0.0, 0.0, 0.0, 0.0, 0.4169650580596226, 0.35712522502518707, 0.31977609475527957, 0.2950788703558871, 0.27795624241578587, 0.3278565142586545, 0.3718649556741534, 0.39947927868857513, 0.42642192325537426], [0.29367080368295195, 0.25, 0.25, 0.25, 0.0, 0.25, 0.2534690834007142, 0.26656376980116075, 0.28721942743545337, 0.32274730112860683, 0.0, 0.0, 0.0, 0.0, 0.0, 0.0, 0.0, 0.0, 0.0, 0.0, 0.0, 0.32139879764473356, 0.2866495373748176, 0.26632581619413065, 0.25338637644479695, 0.25, 0.2776302847051402, 0.3414277887393714, 0.38397340719039036, 0.4144166022214057]]
  in  "pass?":bool=TRUE
  in  "PID gains Radius To Turn":cluster{"(Kc)":dbl, "(Ki)":dbl, "(Kd)":dbl}={"(Kc)"=1.0, "(Ki)"=0.0, "(Kd)"=1e-06}
  in  "PID gains Vel D":cluster{"(Kp)":dbl, "(Ki)":dbl, "(Kd)":dbl}={"(Kp)"=0.25, "(Ki)"=0.0, "(Kd)"=0.001}
  in  "PID gains Angle":cluster{"(Kc)":dbl, "(Ki)":dbl, "(Kd)":dbl}={"(Kc)"=3.0, "(Ki)"=0.0, "(Kd)"=0.002}
  in  "PID gains Angle To Turn":cluster{"(Kc)":dbl, "(Ki)":dbl, "(Kd)":dbl}={"(Kc)"=3.2, "(Ki)"=0.0, "(Kd)"=0.001}
  in  "PID gains Lateral":cluster{"(Kc)":dbl, "(Ki)":dbl, "(Kd)":dbl}={"(Kc)"=1.5, "(Ki)"=0.0, "(Kd)"=0.0015}
  in  "Communication in":refnum<class "Communication.lvclass">
  in  "Frame and Field Size out Ref":T45 {"Detection Frame Out"."robots_blue"."height" format="%+4.3f"; "Detection Frame Out"."robots_blue"."pixel_y" format="%+4.3f"; "Detection Frame Out"."robots_blue"."pixel_x" format="%+4.3f"; "Detection Frame Out"."robots_blue"."orientation" format="%+4.3f"; "Detection Frame Out"."robots_blue"."y" format="%+4.3f"; "Detection Frame Out"."robots_blue"."confidence" format="%4.3f"; "Detection Frame Out"."robots_blue"."x" format="%+4.3f"; "Detection Frame Out"."robots_yellow"."height" format="%+4.3f"; "Detection Frame Out"."robots_yellow"."pixel_y" format="%+4.3f"; "Detection Frame Out"."robots_yellow"."pixel_x" format="%+4.3f"; "Detection Frame Out"."robots_yellow"."orientation" format="%+4.3f"; "Detection Frame Out"."robots_yellow"."y" format="%+4.3f"; "Detection Frame Out"."robots_yellow"."confidence" format="%4.3f"; "Detection Frame Out"."robots_yellow"."x" format="%+4.3f"}
  out "2D Picture":picture
  in  "SSL Referee Game Status Ref":T32 {"Time" format="%<%.3X %x>T"; "Blue Timeout Remaining" format="%<%M:%S>t"; "Yellow Timeout Remaining" format="%<%M:%S>t"; "Time Left" format="%<%M:%S>t"}
  out "GUI Game Status":T32={"Stage"="Post Game", "Command"="Halt", "Time Left"=0.0, "Yellow Team"="RoboIME", "Blue Team"="Warthog Robotics", "Yellow Score"=0, "Blue Score"=5, "Yellow Red Cards"=0, "Blue Red Cards"=0, "Yellow Yellow Cards"=3, "Blue Yellow Cards"=0, "Yellow Timeouts Left"=2, "Blue Timeouts Left"=2, "Yellow Timeout Remaining"=150.0, "Blue Timeout Remaining"=150.0, "Yellow Goalie Id"=3, "Blue Goalie Id"=6, "Time"=timestamp(3779822234.55011 s since 1904-01-01), "Point"={"x"=0.0, "y"=0.0}} {"Time" format="%<%.3X %x>T"; "Blue Timeout Remaining" format="%<%M:%S>t"; "Yellow Timeout Remaining" format="%<%M:%S>t"; "Time Left" format="%<%M:%S>t"}
  # "To execute Test and TestMode(zigzag)\nthe referee command must be Stop"
  # "Score"
  # "Red Cards"
  # "Yellow Cards"
  # "Timeouts Left"
  # "Timeout Remaining"
  # "Goalie ID"
  # "left goal"
  # "right goal"
  # "vision computer"
  # "PID gains vel:\nMakes the current position\napproximate to destiny"
  # "PID gains Angle to Turn:\nAdjust angle while robot\n is turning"
  # "PID gains Radius to Turn:\nAdjust turning radius\nwhile turning"
  # "PID gains Angle:\nAdjust spin angle"
  # "PID gains lateral:\nusado apenas no safe drive"
  # "Score"
  # "Red Cards"
  # "Yellow Cards"
  # "Timeouts Left"
  # "Timeout Remaining"
  # "Goalie ID"
  # "Score"
  # "Red Cards"
  # "Yellow Cards"
  # "Timeouts Left"
  # "Timeout Remaining"
  # "Goalie ID"
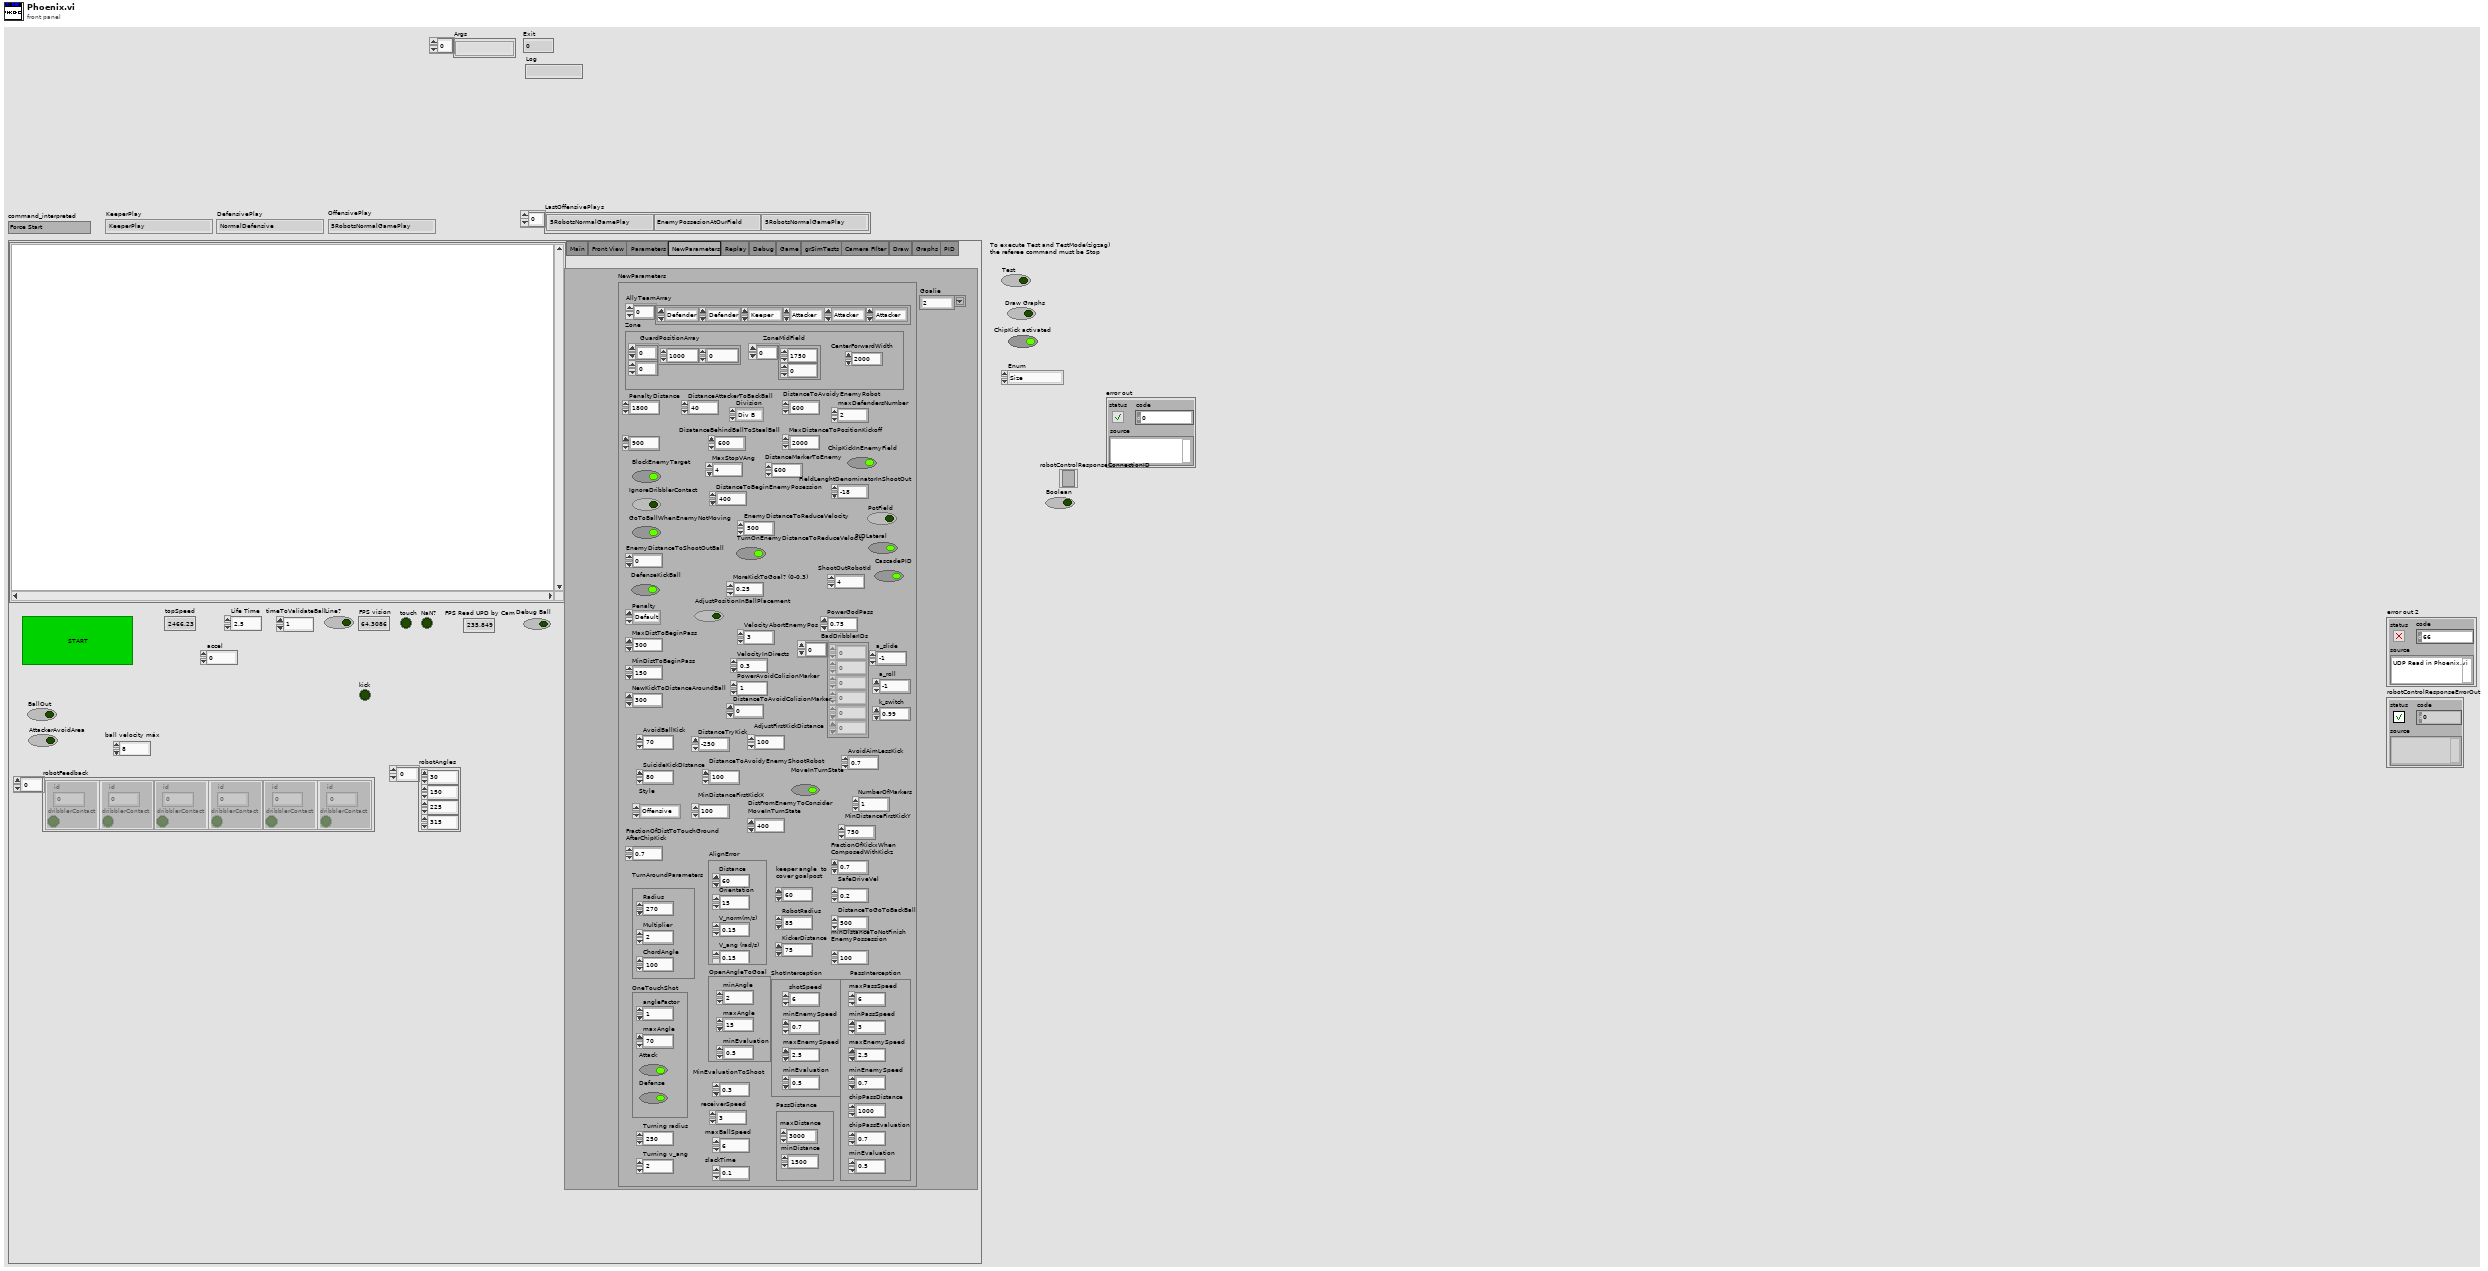
[diagram p1: front panel]
types:
  T1 = typedef "Zone.lvclass/zones.ctl" = enum16{"Field", "LeftSide", "RightSide", "MidField", "LeftForward", "RightForward", "LeftMidField", "RightMidField", "LeftWing", "CenterForward", "RightWing", "Size"}
  T2 = typedef "OffensivePlay.ctl" = enum16{"5RobotsPassGamePlay", "5PreparePassGame", "5RobotsKeeperGame", "KeeperPassToStriker", "5RobotsNormalGamePlay", "PrepareKeeperPass", "ACBPass", "ABCPass", "PrepareTriplePass", "TableWithStriker", "TableWith2ndStrikerPlay", "PrepareDoublePass", "PrepareRollToPass", "SimplePass", "PreparePass", "PassToStriker", "BallOutOfField", "PassTo2ndStriker", "StopOffensive", "Prepare Penalty Enemy", "EnemyPossessionAtEnemyField", "EnemyPossesionAtOurField", "TestPlay", "PreparePenaltyAlly", "KickPenaltyAlly", "PrepareKickoffAlly", "PrepareKickoffEnemy", "IndirectEnemy", "DirectEnemy", "PreparePassInGame1", "NormalGame", "DirectKick", "Pass", "Halt", "Timeout", "PassPlay", "PenaltyEnemy"}
  T3 = typedef "KeeperPlay.ctl" = enum16{"SimpleBallPlacementAlly", "BallPlacementAlly", "BallPlacementEnemy", "ZigZag", "Goto", "NormalGame", "KeeperPlay", "Halt", "Timeout", "PenaltyEnemy", "TestPlay"}
  T4 = typedef "DefensivePlay.ctl" = enum16{"NormalDefensiveWithDuelist", "NormalDefensive", "TestPlay", "Halt", "Timeout", "PenaltyEnemy", "PenaltyAlly", "StopDefensive"}
  T5 = typedef "command_interpreted.ctl" = enum16{"Goal Ally", "Goal Enemy", "Ball Placement Enemy", "Ball Placement Ally", "Normal Half Time", "Extra Time  Break", "Extra Half Time", "None", "Post Game", "PKA Normal Start", "Prepare Kickoff Ally", "PKE Normal Start", "Prepare Kickoff Enemy", "Force Start", "Halt", "Timeout", "Prepare Penalty Ally", "Prepare Penalty Enemy", "PPA NormalStart", "PPE Normal Start", "Indirect Free Ally", "Direct Free Enemy", "Direct Free Ally", "Indirect Free Enemy", "Stop"}
  T6 = typedef "grSimReplacement.ctl" = cluster{"robots":T7[], "ball":T8}
  T7 = typedef "grSim RobotReplacement.ctl" = cluster{"x":dbl, "y":dbl, "dir(degree)":dbl, "yellowteam":bool, "id":u32}
  T8 = typedef "grSim_BallReplacement.ctl" = cluster{"x":dbl, "y":dbl, "vx":dbl, "vy":dbl}
  T9 = cluster{"line_width":u32, "field_length":u32, "field_width":u32, "boundary_width":u32, "referee_width":u32, "goal_width":u32, "goal_depth":u32, "goal_wall_width":u32, "center_circle_radius":u32, "defense_radius":u32, "defense_stretch":u32, "free_kick_from_defense_dist":u32, "penalty_spot_from_field_line_dist":u32, "penalty_line_from_spot_dist":u32}
  T10 = enum32{"Main", "Front View", "Parameters", "NewParameters", "Replay", "Debug", "Game", "grSimTests", "Camera FIlter", "Draw", "Graphs", "PID"}
  T11 = typedef "ParametersFromFile.ctl" = cluster{"UseFiles":bool, "RewriteFilesWithParams":bool}
  T12 = typedef "vision_control.ctl" = cluster{"Local IP:":string, "Server IP:":string, "Port":string}
  T13 = typedef "ComUDP.ctl" = cluster{"UDP GrSim TX":bool, "Address:":string, "Port:":u16}
  T14 = typedef "ComSerial.ctl" = cluster{"Serial TX":bool, "Porta:":refnum<visa-resource-name>}
  T15 = typedef "ComSOS.ctl" = cluster{"UDP SOS TX ":bool, "SOS Port: 2":u16, "SOS Port: ":u16, "SOS Address:":string}
  T16 = typedef "Project.ctl" = enum16{"SSL", "VSS"}
  T17 = typedef "Enviroment.ctl" = enum16{"erForceSimulator", "grSim", "realGame"}
  T18 = enum32{"Invalid", "Standard", "Closed", "Hidden", "Minimized", "Maximized"}
  T19 = typedef "robotDisplayFeedback.ctl" = cluster{"id":dbl, "encoder1":dbl, "encoder2":dbl, "kickCharge":bool, "ballInSensor":bool, "Battery (V)":dbl, "2D Picture":picture, "encoder3":dbl, "encoder4":dbl, "Valid":bool}
  T20 = typedef "PhoenixParameters.ctl" = cluster{"Defensive Marker":enum16{"SecondMostDangerous", "MostDangerous"}, "TimeoutDistanceInX":dbl, "TimeoutDistanceInY":dbl, "DistanceForaStillBall":dbl, "TouchDistance":dbl, "AttackerFarback":dbl, "MinDistToKick":dbl, "Type of Marker":enum16{"Auto", "BlockEnemyPass", "BlockOurGoal"}, "Type of Defense ":enum16{"Barreira", "Manmark"}, "PassAngle":dbl, "KickRange":dbl, "KickForce":dbl, "KickEps":dbl, "KickAngle":dbl, "PassForceMult":dbl, "DistanceToKickingAngle":dbl, "DistanceToBallOut":dbl, "DistanceStop":dbl, "DistanceBehindAttacker":dbl, "Area":enum16{"Circular", "Square"}, "DistanceForPossession":dbl, "DistanceToConsirerRobotArrive":dbl, "DistanceToGoAroundBall":dbl, "DistanceInFrontOfAttacker":dbl, "TimeoutDistanceBetweenRobots":dbl, "MaxOutputAngle":dbl, "MaxOutputXY":dbl, "MaxDeceleration":dbl, "MaxControlIncrement":dbl, "MaxAcceleration":dbl, "AngularToleranceForPossession":dbl, "MaxVelBallToBeginDuelist":dbl, "ZigZagAngle":dbl, "PID gains Vel":cluster{"(Kc)":dbl, "(Ti, min)":dbl, "(Td, min)":dbl}, "Number of Offensive":enum16{"6", "5", "4", "3", "2", "1", "0", "Auto"}, "Shoot Out?":bool, "DefenseAvoidArea":bool, "InvertKick":dbl[], "Simple Pass":bool, "ShootOutForce":dbl, "dtPosEstBall":dbl, "AttkIgnoreBallObst":dbl, "BarrierDist":dbl, "PassReceiver":T21, "GoalieInFrontGoal":dbl, "RollToPass":bool, "PassReceiver":T22, "OldRRT":bool, "Dribbler":bool, "VelNearBall":dbl, "ChipKick Force":dbl, "ForcePass\nInGame":dbl, "bangBangParameters":T23, "BallVelToAbortPass":dbl, "BallVelToFinishPass":dbl, "minDistanceToPass":dbl, "dribbler_rpm":dbl, "AttackerAngle\nToTurnInDegrees":dbl, "AttackerAngle\nToShootInDegrees":dbl, "distToActivateDibbler":dbl, "StopVelocity":dbl, "timeoutToShoot":dbl, "DistanceArea":dbl, "MinDistanceEnemy\nToBallToMark":dbl, "DisableStopAvoidArea":bool, "RRT Parameters":T24, "PID per ID":T25[]}
  T21 = typedef "PassReceiver.ctl" = enum16{"Auto", "2ndStriker", "Striker"}
  T22 = typedef "ChoosePassReceiver.ctl" = enum16{"Striker", "2ndStriker", "Auto"}
  T23 = typedef "bangBangControlParameters.ctl" = cluster{"MaxVSent":dbl, "MaxVNorm":dbl, "MaxVAng":dbl, "VAngCircle":dbl, "LBeginCircle":dbl, "DistToDestOrientation":dbl, "MaxVAngToTurn":dbl, "AtkDistToDestOrientation":dbl, "KepperMaxVSent":dbl, "VelNearEnemy":dbl}
  T24 = typedef "RRTParameters.ctl" = cluster{"threshold":sgl, "Step":sgl, "GoalProb":sgl, "WayPointProb":sgl}
  T25 = typedef "PIDParameters.ctl" = cluster{"PID gains Vel D":cluster{"(Kp)":dbl, "(Ki)":dbl, "(Kd)":dbl}, "PID gains Angle":cluster{"(Kc)":dbl, "(Ki)":dbl, "(Kd)":dbl}, "PID gains Angle To Turn":cluster{"(Kc)":dbl, "(Ki)":dbl, "(Kd)":dbl}, "PID gains Lateral":cluster{"(Kc)":dbl, "(Ki)":dbl, "(Kd)":dbl}}
  T26 = typedef "NewParameters.ctl" = cluster{"PenaltyDistance":dbl, "DistanceAttackerToBackBall":dbl, "Division":enum16{"Div B", "Div A"}, "DistanceToAvoidyEnemyRobot":dbl, "BallPlacementDistance":dbl, "DisatanceBehindBallToStealBall":dbl, "MaxDistanceToPositionKickoff":dbl, "BlockEnemyTarget":bool, "MaxStopVAng":dbl, "DistanceMarkerToEnemy":dbl, "IgnoreDribblerContact":bool, "DistanceToBeginEnemyPosession":dbl, "GoToBallWhenEnemyNotMoving":bool, "EnemyDistanceToReduceVelocity":dbl, "TurnOnEnemyDistanceToReduceVelocity":bool, "EnemyDistanceToShootOutBall":dbl, "DefenseKickBall":bool, "MoreKickToGoal? (0-0.3)":dbl, "ChipKickInEnemyField":bool, "ShootOutRobotId":dbl, "FieldLenghtDenominatorInShootOut":dbl, "AdjustPositionInBallPlacement":bool, "PowerGodPass":dbl, "VelocityAbortEnemyPos":dbl, "MaxDistToBeginPass":dbl, "MinDistToBeginPass":dbl, "VelocityInDirects":dbl, "BadDribblerIDs":i32[], "NewKickToDistanceAroundBall":dbl, "PowerAvoidColisionMarker":dbl, "DistanceToAvoidColisionMarker":dbl, "AvoidBallKick":dbl, "DistanceTryKick":dbl, "SuicideKickDIstance":dbl, "AdjustFirstKickDistance":dbl, "AvoidAimLessKick":dbl, "DistanceToAvoidyEnemyShootRobot ":dbl, "NumberOfMarkers":dbl, "PotField":bool, "PIDLateral":bool, "MinDistanceFirstKickX":dbl, "MinDistanceFirstKickY":dbl, "FractionOfDistToTouchGround\nAfterChipKick":dbl, "FractionOfKickxWhen\nComposedWithKickz":dbl, "Style":T27, "MoveInTurnState":bool, "DistFromEnemyToConsider\nMoveInTurnState":dbl, "CascadePID":bool, "TurnAroundParameters":cluster{"Radius":dbl, "Multiplier":dbl, "ChordAngle":dbl}, "SafeDriveVel":dbl, "DistanceToGoToBackBall":dbl, "minDistanceToNotFinish\nEnemyPossession":dbl, "OneTouchShot":cluster{"angleFactor":dbl, "maxAngle":dbl, "Attack":bool, "Defense":bool}, "OpenAngleToGoal":cluster{"minAngle":dbl, "maxAngle":dbl, "minEvaluation":dbl}, "ShotInterception":cluster{"shotSpeed":dbl, "minEnemySpeed":dbl, "maxEnemySpeed":dbl, "minEvaluation":dbl}, "AllyTeamArray":T28[], "maxDefendersNumber":i32, "Zone":cluster{"GuardPositionArray":dbl[][], "ZoneMidField":dbl[], "CenterForwardWidth":dbl}, "MinEvaluationToShoot":dbl, "PassInterception":cluster{"maxPassSpeed":dbl, "minPassSpeed":dbl, "minEnemySpeed":dbl, "chipPassDistance":dbl, "chipPassEvaluation":dbl, "minEvaluation":dbl, "maxEnemySpeed":dbl}, "PassDistance":cluster{"maxDistance":dbl, "minDistance":dbl}, "receiverSpeed":dbl, "maxBallSpeed":dbl, "slackTime":dbl, "Turning radius":dbl, "Turning v_ang":dbl, "AlignError":cluster{"Distance":dbl, "Orientation":dbl, "V_norm(m/s)":dbl, "V_ang (rad/s)":dbl}, "RobotRadius":dbl, "KickerDistance":dbl, "keeper angle  to cover goalpost":dbl, "a_slide":dbl, "a_roll":dbl, "k_switch":dbl, "Penalty":u16}
  T27 = typedef "Style.ctl" = enum16{"Insanity", "Offensive", "Defensive"}
  T28 = typedef "AllyTeam.ctl" = enum16{"Keeper", "Defender", "Attacker"}
  T29 = typedef "ReplayControls.ctl" = cluster{"Slide":dbl, "Enable":bool, "FPS":dbl, "On":bool, "Play":bool, "CopyFile":bool, "CopyFilePathRelativeToLogFolder":string, "ReadFromFile":bool, "ReadPathRelativeToLogFolder":string, "FrameBufferSize":dbl, "Speed":dbl}
  T30 = typedef "roles.ctl" = enum16{"SimpleBallPlacement", "BallPlacementAllyPasser", "BallPlacementAllyReceiver", "BallPlacementEnemy", "5Robots5th", "PassBestReceiver", "5Robots4th", "5Robots3rd", "5Robots2nd", "5Robots1st", "PassBestRobot", "WaitPass", "ABCThirdKicker", "ABCFirstKicker", "ABCSecondKicker", "Tabler", "TableFinalizer", "PrepareRollToPassRoller", "PrepareRollToPassReceiver", "SimplePassRoll", "SimplePassRollReceiver", "PenaltyDefense", "PreparePassReceiver 2", "PreparePassReceiver 1", "PassObserver", "Timeout", "Goto", "ZigZag", "None", "BallOutOfField", "DefenderArea", "Duelist", "AttackerStop", "FollowAttacker", "KeeperRole", "KickPenalty", "AttackerAimGoal", "AttackerBlock", "Marker", "Halt", "Shoot", "PassKicker", "PassReceiver", "TestRole", "PenaltyAttacker"}
  T31 = typedef "tactics.ctl" = enum16{"GoToBallPlacementPosition", "PlaceBall", "GoToBallPlacement", "5Robots", "BallPlacementEnemy", "ReceivePassInFuturePoint", "Roller", "PrepareRollToPassRollerGoTo", "PrepareRollToPassReceiverGoTo", "WaitRoll", "PositionToRoll", "PenaltyAttacker", "PassObserver", "PenaltyDefense", "TableReceiverTactic", "Test", "DefendGoal", "Marker", "FollowAttacker", "DefendArea", "Shoot", "AttackerAimGoal", "AttackerBallOutOfField", "AttackerBlock", "AttackerStop", "Duelist", "Halt", "ZigZag", "GoTo", "Timeout", "KickToBestRobot", "KickToPassReceiver", "PositionToReceivePass", "WaitPass", "GoToTarget"}
  T32 = typedef "SSL Referee Game Status.ctl" = cluster{"Stage":string, "Command":string, "Time Left":dbl, "Yellow Team":string, "Blue Team":string, "Yellow Score":u32, "Blue Score":u32, "Yellow Red Cards":u32, "Blue Red Cards":u32, "Yellow Yellow Cards":u32, "Blue Yellow Cards":u32, "Yellow Timeouts Left":u32, "Blue Timeouts Left":u32, "Yellow Timeout Remaining":dbl, "Blue Timeout Remaining":dbl, "Yellow Goalie Id":u32, "Blue Goalie Id":u32, "Time":timestamp, "Point":cluster{"x":sgl, "y":sgl}}
  T33 = typedef "RobotModelTestState.ctl" = cluster{"current sample":i32, "V0":dbl, "Vf":dbl, "progress":dbl, "current state":i32, "est_vel":dbl, "V_sent":dbl, "crash cases":bool}
  T34 = typedef "testMode.ctl" = enum16{"2DbangbangTest", "KickForce", "TimeTrajectory", "ZigZag", "KickValue", "VelocityPlanning", "RobotModel", "RobotModelStateSpace", "CorumbaTest", "TurnTest"}
  T35 = typedef "RobotModelReplacementTest.ctl" = cluster{"grSIM replacement":T6, "replace active":bool, "TestParameters":cluster{"Start":bool, "V_sent(not used\nmore)":dbl, "id":i32, "Samples":dbl, "V_sample":dbl, "delta":dbl, "Test number":dbl}, "Dest_array":cluster{"dest_x":dbl, "dest_y":dbl, "dest_orientation":dbl, "dest_vel":dbl}[][], "replaceBall":bool, "ballVelocity":dbl, "timeoutKick":dbl, "KickValueTest":T36, "StateSpaceTestParameters":cluster{"Start":bool, "uMaxPos":dbl, "frequency":i32, "Samples":dbl, "uMinPos":dbl, "holdingFrequency":dbl, "uMaxAngle":dbl, "uMinAngle":dbl, "id":dbl}}
  T36 = typedef "KickValuetest.ctl" = cluster{"ForceValue":T37, "BallValue":T38, "Samples":dbl, "Start":bool, "id":i32, "RobotStopKick":bool}
  T37 = typedef "Game.lvclass/KickValue.ctl" = cluster{"delta_kick":dbl, "kick_min":dbl, "kick_max":dbl}
  T38 = typedef "Game.lvclass/BallValue.ctl" = cluster{"delta_ball":dbl, "v_min_ball":dbl, "v_max_ball":dbl}
  T39 = typedef "velocityPlanningState.ctl" = cluster{"est_vel":dbl, "dist_to_(Dest/L)":dbl, "V0_model":dbl, "max_dist_to_break":dbl, "v_sent":dbl, "traj_state":T40}
  T40 = typedef "trajectoryState.ctl" = enum16{"stop", "replace", "circle", "line", "turn"}
  T41 = typedef "Game.lvclass/kickForceTestState.ctl" = cluster{"currentKickForce":dbl, "targetBallVelocity":dbl, "est_bal_vell":dbl, "sample":dbl, "state":T42}
  T42 = typedef "Game.lvclass/KickForceEnum.ctl" = enum16{"Finish", "Velball", "GoToNextKickForce", "WaitBall", "KickBall", "ReplaceBall"}
  T43 = typedef "Estimadores.ctl" = enum16{"Variable2ndDerivate", "4thDerivate", "2ndDerivate", "Nenhum", "Simples", "Kalman", "Kalman2023"}
  T44 = typedef "DrawTargets.ctl" = cluster{"Attacker":bool, "Striker":bool, "Goalie":bool, "Defender":bool, "kick":bool, "Est Ball":bool, "Est Robot":bool, "Path S":bool, "Path C":bool, "Dngr.Enemy":bool, "2nd Striker":bool}
  T45 = typedef "SSL Field State.ctl" = cluster{"Detection Frame Out":T46, "Field Size Out":cluster{"line_width":u32, "field_length":u32, "field_width":u32, "boundary_width":u32, "referee_width":u32, "goal_width":u32, "goal_depth":u32, "goal_wall_width":u32, "center_circle_radius":u32, "defense_radius":u32, "defense_stretch":u32, "free_kick_from_defense_dist":u32, "penalty_spot_from_field_line_dist":u32, "penalty_line_from_spot_dist":u32}, "Received Time Stamp":timestamp}
  T46 = typedef "SSL Detection Frame.ctl" = cluster{"frame_number":u32, "t_capture":dbl, "t_sent":dbl, "camera_id":u32, "robots_yellow":T47[], "robots_blue":T47[], "balls":T49[], "Valid":bool, "Time Stamp":timestamp, "New":bool, "Initialized":bool}
  T47 = typedef "SSL Detection Robot.ctl" = cluster{"x":sgl, "robot_id":u32, "confidence":sgl, "y":sgl, "orientation":sgl, "pixel_x":sgl, "pixel_y":sgl, "height":sgl, "Valid":bool, "Time Stamp":timestamp, "x_k|k":T48, "Pk|k":T48, "Previous Time Stamp":timestamp, "R":T48, "vx":dbl, "vy":dbl, "vang":dbl}
  T48 = typedef "NI_Matrix.lvlib/RealMatrix.ctl" = dbl[][]
  T49 = typedef "SSL Detection Ball.ctl" = cluster{"x":sgl, "area":u32, "confidence":sgl, "y":sgl, "z":sgl, "pixel_x":sgl, "pixel_y":sgl, "Valid":bool, "Time Stamp":timestamp, "x_k|k":T48, "Pk|k":T48, "Id":u32, "Previous Time Stamp":timestamp, "R":T48, " vx":sgl, "vy":dbl, "vz":dbl, " ax":sgl, "ay":dbl, "az":dbl}
  T50 = typedef "Vision.lvclass/SSL_BallModelStraightTwoPhase.ctl" = cluster{"acc_slide":dbl, "acc_roll":dbl, "k_switch":dbl}
  T51 = typedef "ReplayInfo.ctl" = cluster{"ByteArrayFromVision":u8[], "TimeStampSampledInReplay":string, "ByteArrayFromReferee":u8[], "AllyRobotExtraInfoArray":T52[], "EnemyRobotExtraInfoArray":T52[]}
  T52 = typedef "RobotExtraInfo.ctl" = cluster{"est_vx":dbl, "est_vy":dbl, "id":dbl}
  T53 = typedef "AI Input.ctl" = cluster{"our_robots":T54[], "enemy_robots":T54[], "balls":T63[], "geometry":T64, "IA Judge":T65, "Received Timestamp":timestamp, "Events":T67}
  T54 = typedef "AI Robot.ctl" = cluster{"id":u32, "function":T55, "x":dbl, "y":dbl, "orientation":dbl, "v_tangent":dbl, "v_normal":dbl, "v_ang":dbl, "kick_x":dbl, "kick_z":dbl, "dribble":bool, "Timestamp":timestamp, "estimatives":T56, "dest_x_kick":dbl, "dest_y_kick":dbl, "Gap Coord":dbl[], "States":T57, "Path ":dbl[][], "Path  Smooth":dbl[][], "Dest":T58, "vx_desired":dbl, "vy_desired":dbl, "slowBehavior":bool, "VSSStates":T60, "robotKickState":T61, "role":T30, "x_k|k":T48, "driveMode":T62}
  T55 = typedef "Functions Enum.ctl" = enum16{"2nd Striker", "Attacker", "Goalie", "Defender", "Striker", "Goto 0", "Dummy", "Kicker", "ZigZag 0", "ZigZag 1", "ZigZag 2", "ZigZag 3", "ZigZag 4", "ZigZag 5", "ZigZag 6", "ZigZag 7", "ZigZag 8", ""}
  T56 = typedef "estimatives.ctl" = cluster{"est_v_tangent":dbl, "est_v_normal":dbl, "est_vx":dbl, "est_vy":dbl, "Pos Robot Est":dbl[], "est_v_ang":dbl}
  T57 = typedef "AttackerStates.ctl" = enum16{"Pass", "GoToTangent", "BallGetting", "GoToKick", ""}
  T58 = typedef "PathDests.ctl" = T59[]
  T59 = typedef "PathDest.ctl" = cluster{"dest_x":dbl, "dest_y":dbl, "dest_orientation":dbl, "dest_vel":dbl}
  T60 = typedef "VSSAttackerStates.ctl" = enum16{"Pass", "GoToTangent", "BallGetting", "GoToKick", "Rotate anti-clockwise", "Rotate Clockwise", ""}
  T61 = typedef "robotKickToStates.ctl" = enum16{"shootFromDirect", "avoidCollideBall", "goToBackBall", "none", "walk", "turn", "turnAntiClockWise", "turnClockwise", "oldKickToShoot", "oldKickToGoToBackBall", "shoot"}
  T62 = typedef "driveMode.ctl" = enum16{"Fast", "SafeDrive"}
  T63 = typedef "AI Ball.ctl" = cluster{"x":dbl, "y":dbl, "timestamp":timestamp, "Vel_x":dbl, "Vel_y":dbl, "Pos Bola Est":dbl[], "Valid":bool, "z":dbl, "Vel_z":dbl, "Accel_x":dbl, "Accel_y":dbl}
  T64 = typedef "Field Size.ctl" = cluster{"line_width":u32, "field_length":u32, "field_width":u32, "boundary_width":u32, "referee_width":u32, "goal_width":u32, "goal_depth":u32, "goal_wall_width":u32, "center_circle_radius":u32, "defense_radius":u32, "defense_stretch":u32, "free_kick_from_defense_dist":u32, "penalty_spot_from_field_line_dist":u32, "penalty_line_from_spot_dist":u32}
  T65 = typedef "AI Judge.ctl" = cluster{"stage":string, "command":string, "our_goalie_id":dbl, "enemy_goalie_id":dbl, "command enum":T66, "Time":enum16{"Azul", "Amarelo"}, "Point":cluster{"x":sgl, "y":sgl}}
  T66 = typedef "Command Enum.ctl" = enum16{"Halt", "Stop", "Force Start", "PKA Normal Start", "Prepare Kickoff Ally", "PKE Normal Start", "Prepare Kickoff Enemy", "Prepare Penalty Ally", "PPA Normal Start", "Prepare Penalty Enemy", "PPE Normal Start", "Direct Free Enemy", "Direct Free Ally", "Indirect Free Enemy", "Indirect Free Ally", "Timeout Enemy", "Timeout Ally", "Goal Enemy", "Goal Ally", "Ball Placement Enemy", "Ball Placement Ally", "Normal Half Time", "Extra Time Break", "Extra Half Time", "None", "Post Game"}
  T67 = typedef "Events.ctl" = cluster{"Touch":bool, "Ball out":bool, "id touch":dbl, "Ball out of \nVision":bool, "Ball inside \nGoalie area":bool, "Robot not responding":bool, "Robots responding status":dbl[], "Enemy Ball \nPossession":bool, "Pass State":bool, "id end of pass":dbl, "Kick":bool, "Id ini Possession":dbl, "Ball Possesion":bool, "Id Possesion":dbl, "Direct Kick":bool, "2nd Strk Ativo":bool}
  T68 = typedef "MainGameConfigs.ctl" = cluster{"SSL UDP RX":T12, "RefBox UDP RX":T12, "Com UDP":T13, "Command":string, "Goalie":string, "Side":enum16{"Esquerdo", "Direito"}, "Team":enum16{"Azul", "Amarelo"}}
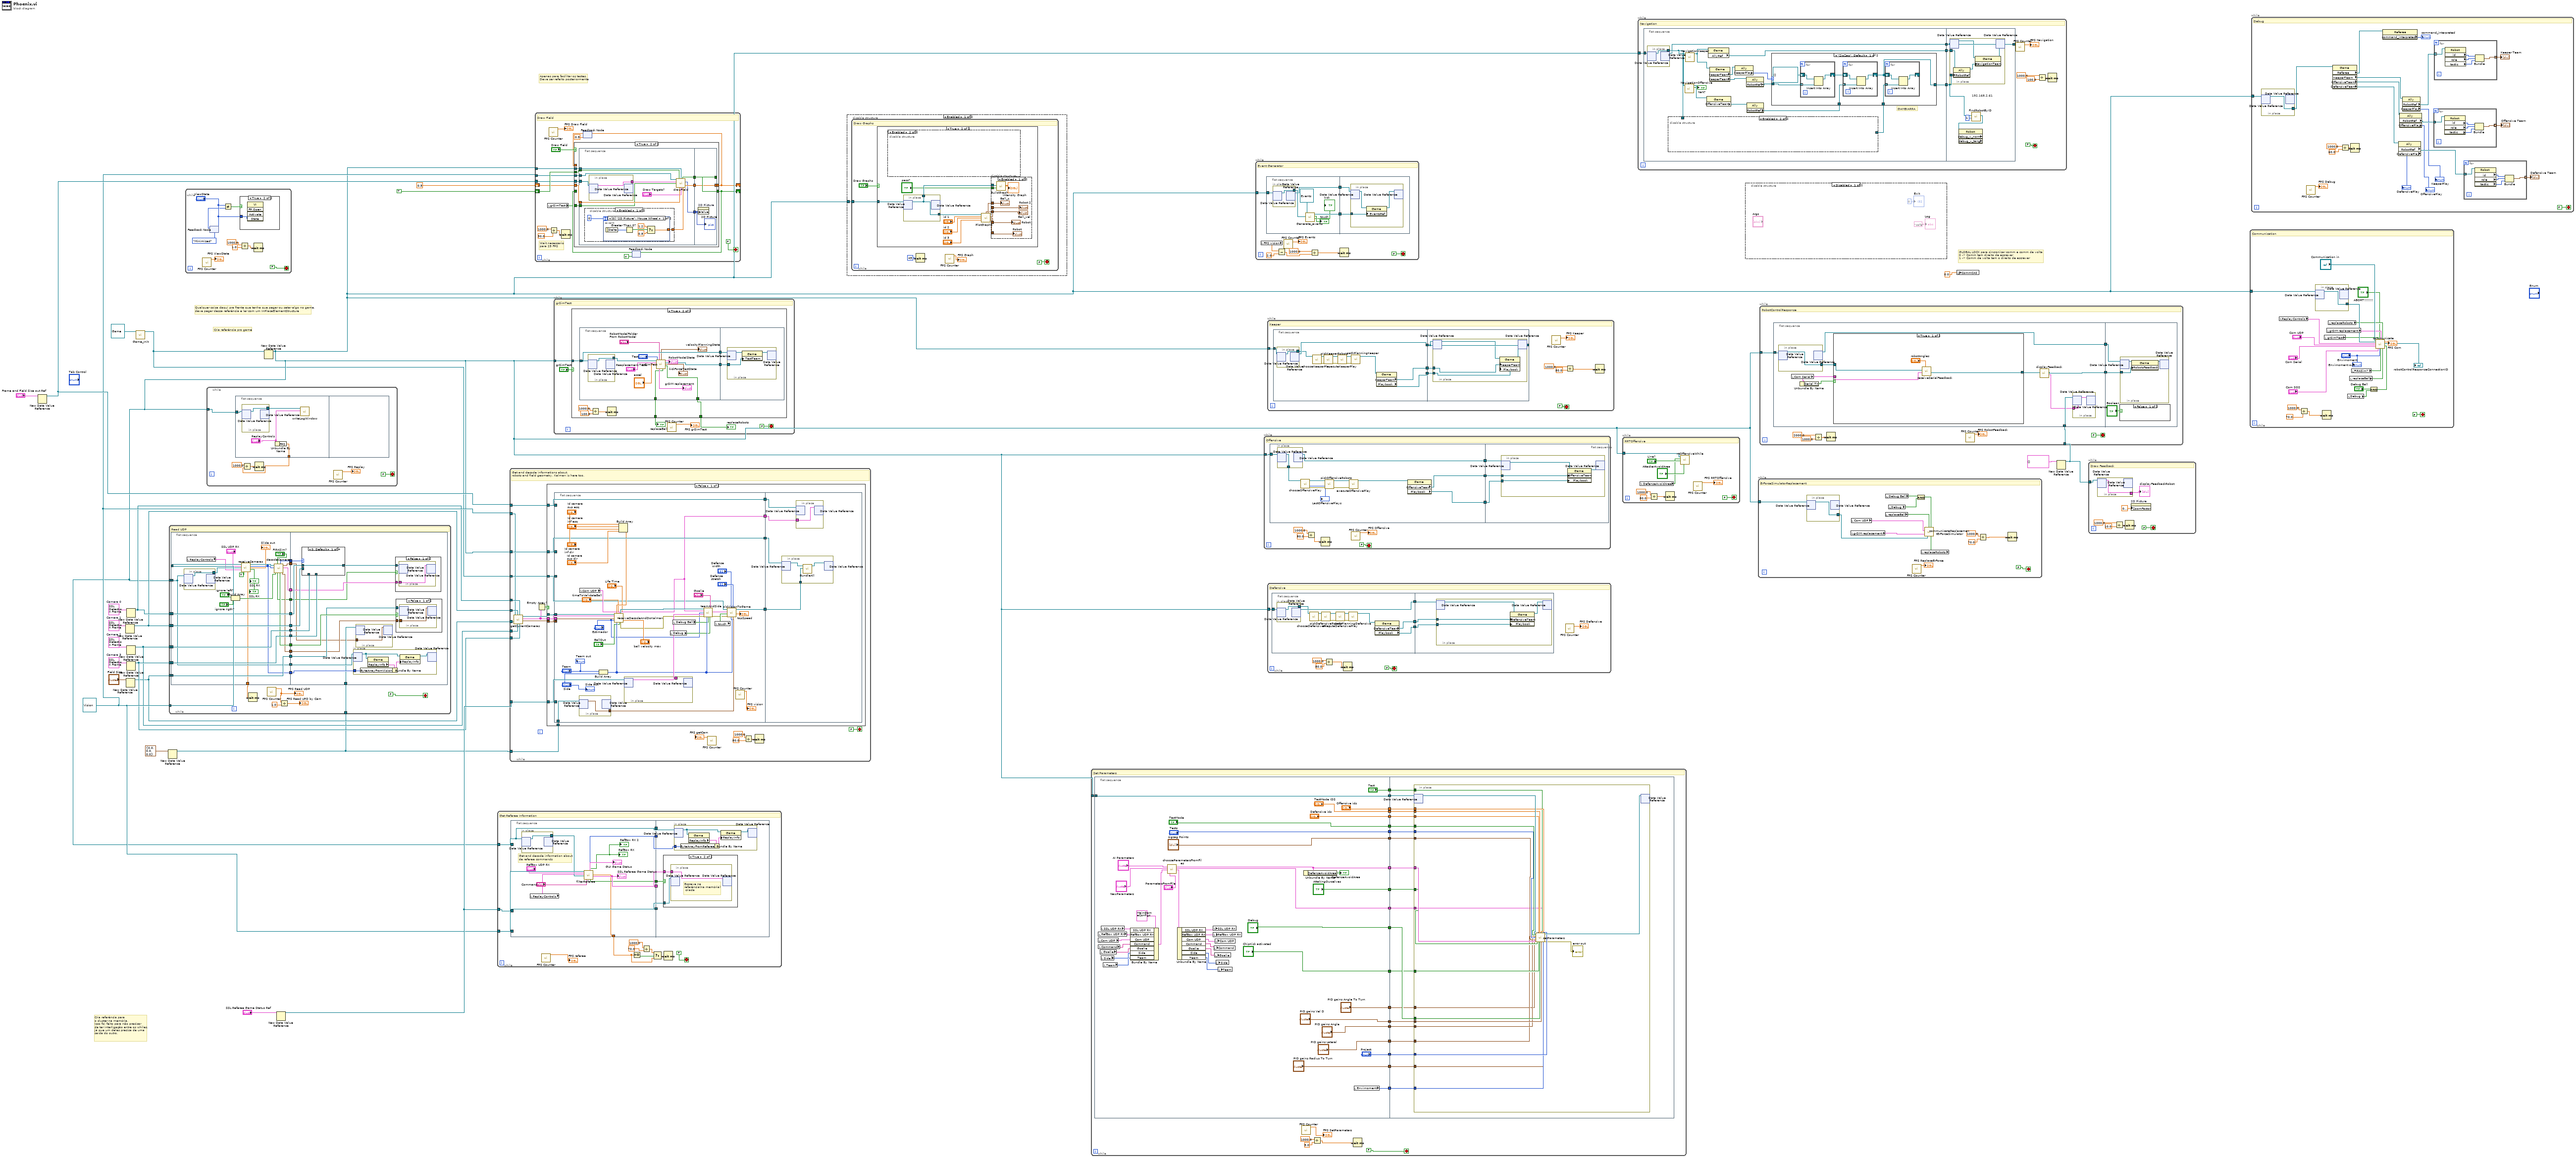
[diagram p0: block diagram]
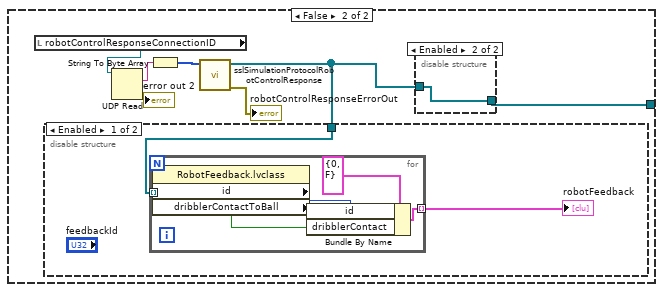
[diagram p9: hidden frame]
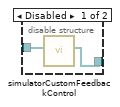
[diagram p10: hidden frame]
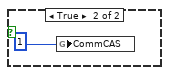
[diagram p12: hidden frame]
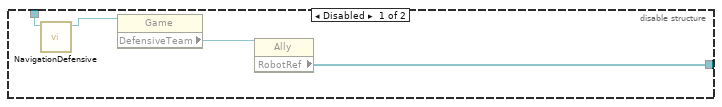
[diagram p15: hidden frame]
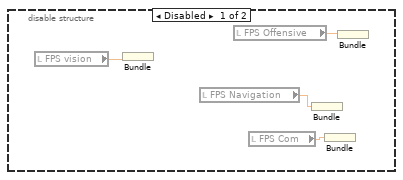
[diagram p18: hidden frame]
diagram:
  w15 = T46 {"frame_number"=0, "t_capture"=0.0, "t_sent"=0.0, "camera_id"=0, "robots_yellow"=[], "robots_blue"=[], "balls"=[], "Valid"=FALSE, "Time Stamp"=timestamp(0 s since 1904-01-01), "New"=FALSE, "Initialized"=FALSE}  # Camera 3
  w16 = T46 {"frame_number"=0, "t_capture"=0.0, "t_sent"=0.0, "camera_id"=0, "robots_yellow"=[], "robots_blue"=[], "balls"=[], "Valid"=FALSE, "Time Stamp"=timestamp(0 s since 1904-01-01), "New"=FALSE, "Initialized"=FALSE}  # Camera 2
  w17 = T46 {"frame_number"=0, "t_capture"=0.0, "t_sent"=0.0, "camera_id"=0, "robots_yellow"=[], "robots_blue"=[], "balls"=[], "Valid"=FALSE, "Time Stamp"=timestamp(0 s since 1904-01-01), "New"=FALSE, "Initialized"=FALSE}  # Camera 1
  w18 = T46 {"frame_number"=0, "t_capture"=0.0, "t_sent"=0.0, "camera_id"=0, "robots_yellow"=[], "robots_blue"=[], "balls"=[], "Valid"=FALSE, "Time Stamp"=timestamp(0 s since 1904-01-01), "New"=FALSE, "Initialized"=FALSE}  # Camera 0
  w19 = refnum<class "Vision.lvclass"> refnum ("Vision")
  # "GLOBAL LOCK para sincronizar comm e comm de volta\n0 -> Comm tem direito de escrever\n1 -> Comm de volta tem o direito de escrever"
  # "Apenas para facilitar os testes.\nDeve ser refeito posteriormente"
  # "Qualquer coisa daqui pra frente que tenha que pegar ou setar algo no game,\ndeve pegar dessa referência e ler com um InPlaceElementStructure"
  # "Cria referência pro game"
  # "Cria referência para\no cluster na memória.\nIsso foi feito para não precisar\nde ter interligação entre os whiles,\njá que um deles precisa de uma\nsaída do outro."
  n1 = New Data Value Reference(data value="Frame and Field Size out Ref") -> (data value reference=w20:refnum<data-value>)  [unwired: 1 in, 1 out]
  n2 = New Data Value Reference(data value=w17) -> (data value reference=w10:refnum<data-value>)  [unwired: 1 in, 1 out]
  n3 = New Data Value Reference(data value="Field Size") -> (data value reference=w9:refnum<data-value>)  [unwired: 1 in, 1 out]
  n4 = New Data Value Reference(data value=w18) -> (data value reference=w11:refnum<data-value>)  [unwired: 1 in, 1 out]
  n5 = New Data Value Reference(data value=w16) -> (data value reference=w12:refnum<data-value>)  [unwired: 1 in, 1 out]
  n6 = New Data Value Reference(data value=w15) -> (data value reference=w13:refnum<data-value>)  [unwired: 1 in, 1 out]
  n7 = call "Game_Init.vi"("object in"=refnum<class "Game.lvclass"> refnum ("Game")) -> ("object out"=w3:refnum<class "Game.lvclass">)  [unwired: 17 in, 1 out]
  n8 = New Data Value Reference(data value=T50 {"acc_slide"=0.0, "acc_roll"=0.0, "k_switch"=0.0} ("SSL_BallModelStraightTwoPhase")) -> (data value reference=w1:refnum<data-value>)  [unwired: 1 in, 1 out]
  n9 = while {
    stop <- FALSE stop-if-true
    n10 = call "FPS Counter.vi"() -> ("FPS"=→"FPS ViewState":dbl)  [unwired: 11 in]
    n11 = feedback-in #1("ViewState") -> ()
    n12 = feedback #1(T18."Minimized" ("ViewState")) -> (w28:T18)
    n13 = Not Equal?(x="ViewState", y=w28) -> (x != y?=w27:bool)
    n14 = case shown="True" w27 {
      tunnel: "ViewState" -> [_ w35]
      frame False {
      }
      frame True {
        n15 = invoke class="VI" method="FP.Open"("State"=w35) -> ()  [unwired: 4 in, 5 out]
      }
    }
    n16 = Divide(x=1000.0, y=1.0) -> (x/y=w31:dbl)
    n17 = Wait (ms)(milliseconds to wait=w31) -> ()  [unwired: 1 out]
  }
  n18 = New Data Value Reference(data value=w3) -> (data value reference=w8:refnum<data-value>)  [unwired: 1 in, 1 out]
  n19 = while {
    tunnel: w19 -> [w61]
    tunnel: w9 -> [w60]
    tunnel: w13 -> [w58]
    tunnel: w11 -> [w56]
    tunnel: w10 -> [w54]
    tunnel: w12 -> [w52]
    tunnel: w8 -> [w42]
    tunnel: w1 -> [w37]
    stop <- FALSE stop-if-true
    # "Read UDP"
    n20 = flat-sequence {
      tunnel: w61 -> [w87]
      tunnel: w60 -> [w80]
      tunnel: [w85] -> w59
      tunnel: w58 -> [w85]
      tunnel: [w84] -> w57
      tunnel: w56 -> [w84]
      tunnel: [w83] -> w55
      tunnel: w54 -> [w83]
      tunnel: [w82] -> w53
      tunnel: w52 -> [w82]
      tunnel: [w81] -> w51
      tunnel: [w80] -> w50
      tunnel: [w79] -> w49
      tunnel: [w78] -> w48
      tunnel: [w72] -> w47
      tunnel: [w77] -> w46
      tunnel: w42 -> [w69]
      tunnel: [w69] -> w41
      tunnel: [w70] -> w40
      tunnel: [w66] -> w39
      tunnel: [w62] -> w36
      tunnel: w59 -> [w100]
      tunnel: w57 -> [w103]
      tunnel: w55 -> [w102]
      tunnel: w53 -> [w101]
      tunnel: w51 -> [w98]
      tunnel: w50 -> [w97]
      tunnel: w49 -> [w96]
      tunnel: w48 -> [w95]
      tunnel: w47 -> [w94]
      tunnel: w46 -> [w93]
      tunnel: w41 -> [w92]
      tunnel: w40 -> [w91]
      tunnel: w37 -> [w90]
      tunnel: w36 -> [w89]
      frame #0 {
        n21 = in-place {
          in-place-border: [w88] -> w68
          n22 = in-place-dvr #2(w69) -> (w88:refnum<class "Game.lvclass">)  [unwired: 1 out]
          n23 = in-place-dvr #2() -> ()  [unwired: 1 in, 2 out]
        }
        n24 = local read "ReplayControls"() -> (w64:T29)
        n25 = Build Array("ignore left?", "ignore rigth?") -> (w74:bool[])
        n26 = call "receiveCameras.vi"("Vision in"=w87, "SSL UDP RX"="SSL UDP RX", "Game"=w68, "ReplayControls"=w64, "vision?"=TRUE) -> ("Vision out"=w86:refnum<class "Vision.lvclass">, "data camera out"=w70:u8[], "Slide out"=→"Slide out":dbl, "RX"=→"SSL RX" →"SSL RX":bool, "delay"=w66:dbl)  [unwired: 5 in, 1 out]
        n27 = call "decodeCameras.vi"("FIRASim?"="FIRASim?", "Ignore left/rigth?"=w74, "unsigned byte array"=w70, "Vision in"=w86) -> ("Field Size"=w79:T9, "Detection Frame"=w72:T46, "SSL_BallModelStraightTwoPhase"=w62:T50, "Empty Field Size?"=w81:bool, "camera_id"=w78:u32, "Empty Information?"=w77:bool)  [unwired: 1 in, 1 out]
      }
      frame #1 {
        n28 = case shown="0, Default" w95 {
          tunnel: [w105 w106 w107 w108] -> w99
          tunnel: w103 -> [w105 _ _ _]
          tunnel: w102 -> [_ w106 _ _]
          tunnel: w101 -> [_ _ w107 _]
          tunnel: w100 -> [_ _ _ w108]
          frame 0, Default {
          }
          frame 1 {
          }
          frame 2 {
          }
          frame 3 {
          }
        }
        n29 = in-place {
          in-place-border: w91 -> [w110]
          n30 = in-place-dvr #3(w92) -> (w112:refnum<class "Game.lvclass">)  [unwired: 1 out]
          n31 = property class="Game"(reference=w112) -> ("ReplayInfo"=w111:T51)  [unwired: 1 in, 2 out]
          n32 = Bundle By Name(cluster=w111, "ByteArrayFromVision"=w110) -> (w109:T51)
          n33 = property class="Game"(reference=w112, "ReplayInfo"=w109) -> (reference out=w113:refnum<class "Game.lvclass">)  [unwired: 1 in, 1 out]
          n34 = in-place-dvr #3(w113) -> ()  [unwired: 2 out]
        }
        n35 = in-place {
          in-place-border: w89 -> [w104]
          n36 = in-place-dvr #4(w90) -> ()  [unwired: 2 out]
          n37 = in-place-dvr #4(w104) -> ()  [unwired: 2 out]
        }
        n38 = case shown="False" w93 {
          tunnel: w99 -> [w118 _]
          tunnel: w94 -> [w117 _]
          frame False {
            n39 = in-place {
              in-place-border: w117 -> [w119]
              n40 = in-place-dvr #5(w118) -> ()  [unwired: 2 out]
              n41 = in-place-dvr #5(w119) -> ()  [unwired: 2 out]
            }
          }
          frame True {
          }
        }
        n42 = case shown="False" w98 {
          tunnel: w97 -> [w115 _]
          tunnel: w96 -> [w114 _]
          frame False {
            n43 = in-place {
              in-place-border: w114 -> [w116]
              n44 = in-place-dvr #6(w115) -> ()  [unwired: 2 out]
              n45 = in-place-dvr #6(w116) -> ()  [unwired: 2 out]
            }
          }
          frame True {
          }
        }
      }
    }
    n46 = Wait (ms)(milliseconds to wait=w39) -> ()  [unwired: 1 out]
    n47 = call "FPS Counter.vi"() -> ("FPS"=w45:dbl)  [unwired: 11 in]
    "FPS Read UDP" <- w45
    n48 = Divide(x=w45, y=1.0) -> (x/y=→"FPS Read UPD by Cam":dbl)
  }
  n49 = while {
    tunnel: w8 -> [w123]
    stop <- FALSE stop-if-true
    n50 = flat-sequence {
      tunnel: [w127] -> w120
      tunnel: w123 -> [w128]
      frame #0 {
        n51 = in-place {
          in-place-border: [w130] -> w129
          n52 = in-place-dvr #7(w128) -> (w130:refnum<class "Game.lvclass">)  [unwired: 1 out]
          n53 = in-place-dvr #7() -> ()  [unwired: 1 in, 2 out]
        }
        n54 = Unbundle By Name("ReplayControls") -> ("FPS"=w127:dbl)
        n55 = call "writeLogWindow.vi"("ReplayControls"="ReplayControls", "Game in"=w129) -> ()  [unwired: 8 in, 2 out]
      }
      frame #1 {
      }
    }
    n56 = Divide(x=1000.0, y=w120) -> (x/y=w125:dbl)
    n57 = Wait (ms)(milliseconds to wait=w125) -> ()  [unwired: 1 out]
    n58 = call "FPS Counter.vi"() -> ("FPS"=→"FPS Replay":dbl)  [unwired: 11 in]
  }
  n59 = New Data Value Reference(data value="SSL Referee Game Status Ref") -> (data value reference=w24:refnum<data-value>)  [unwired: 1 in, 1 out]
  n60 = while {
    tunnel: w19 -> [w146]
    tunnel: w24 -> [w142]
    tunnel: w8 -> [w136]
    stop <- FALSE stop-if-true
    # "Get Referee Information"
    n61 = flat-sequence {
      tunnel: w146 -> [w158]
      tunnel: [w156] -> w143
      tunnel: w142 -> [w156]
      tunnel: [w155] -> w141
      tunnel: [w153] -> w138
      tunnel: [w152] -> w137
      tunnel: w136 -> [w149]
      tunnel: [w151] -> w132
      tunnel: [w149] -> w135
      tunnel: w143 -> [w165]
      tunnel: w141 -> [w164]
      tunnel: w138 -> [w163]
      tunnel: w137 -> [w161]
      tunnel: w135 -> [w162]
      frame #0 {
        # "Get and decode information about\nde referee commands"
        n62 = in-place {
          in-place-border: [w160] -> w150
          n63 = in-place-dvr #8(w149) -> (w160:refnum<class "Game.lvclass">)  [unwired: 1 out]
          n64 = in-place-dvr #8() -> ()  [unwired: 1 in, 2 out]
        }
        n65 = local read "ReplayControls"() -> (w148:T29)
        n66 = call "filterReferee.vi"("Vision in"=w158, "RefBox UDP RX"="RefBox UDP RX", "ReplayControls"=w148, "Game"=w150, "Command"="Command") -> ("RX"=→"RefBox RX" →"RefBox RX 2":bool, "writeInReference"=w153:bool, "GUI Game Status"=→"GUI Game Status":T32, "delay"=w151:dbl, "SSL Referee Game Status"=w155:T32, "data camera out"=w152:u8[])  [unwired: 7 in, 2 out]
        "SSL Referee Game Status" <- w155
      }
      frame #1 {
        n67 = case shown="True" w163 {
          tunnel: w165 -> [_ w172]
          tunnel: w164 -> [_ w171]
          frame False {
          }
          frame True {
            n68 = in-place {
              in-place-border: w171 -> [w173]
              # "Escreve na\nreferência(na memória)\n criada"
              n69 = in-place-dvr #9(w172) -> ()  [unwired: 2 out]
              n70 = in-place-dvr #9(w173) -> ()  [unwired: 2 out]
            }
          }
        }
        n71 = in-place {
          in-place-border: w161 -> [w167]
          n72 = in-place-dvr #10(w162) -> (w169:refnum<class "Game.lvclass">)  [unwired: 1 out]
          n73 = property class="Game"(reference=w169) -> ("ReplayInfo"=w168:T51)  [unwired: 1 in, 2 out]
          n74 = Bundle By Name(cluster=w168, "ByteArrayFromReferee"=w167) -> (w166:T51)
          n75 = property class="Game"(reference=w169, "ReplayInfo"=w166) -> (reference out=w170:refnum<class "Game.lvclass">)  [unwired: 1 in, 1 out]
          n76 = in-place-dvr #10(w170) -> ()  [unwired: 2 out]
        }
      }
    }
    n77 = call "FPS Counter.vi"() -> ("FPS"=→"FPS referee":dbl)  [unwired: 11 in]
    n78 = Equal To 0?(x=w132) -> (x = 0?=w134:bool)
    n79 = Divide(x=1000.0, y=70.0) -> (x/y=w133:dbl)
    n80 = Select(t=w133, s=w134, f=w132) -> (s? t:f=w131:dbl)
    n81 = Wait (ms)(milliseconds to wait=w131) -> ()  [unwired: 1 out]
  }
  n82 = while {
    tunnel: w19 -> [w183]
    tunnel: w24 -> [w192]
    tunnel: w8 -> [w189]
    tunnel: w20 -> [w190]
    tunnel: w3 -> [w191]
    tunnel: w13 -> [w187]
    tunnel: w12 -> [w186]
    tunnel: w11 -> [w184]
    tunnel: w10 -> [w185]
    tunnel: w9 -> [w188]
    tunnel: w1 -> [w174]
    stop <- FALSE stop-if-true
    # "Get and decode informations about\nrobots and field geometry. Kalman is here too."
    n83 = call "getCurrentCameras.vi"("Camera 3"=w187, "Camera 0"=w184, "Camera 2"=w186, "Camera 1"=w185, "Field Size"=w188, "Vision in"=w183) -> ("Field Size out"=w181:T9, "NewCameras"=w180:T46[], "Vision out"=w182:refnum<class "Vision.lvclass">)  [unwired: 2 in, 1 out]
    n84 = Empty Array?(array=w180) -> (empty?=w175:bool)
    n85 = case shown="False" w175 {
      tunnel: w192 -> [w201 _]
      tunnel: w191 -> [w200 _]
      tunnel: w190 -> [w199 _]
      tunnel: w189 -> [w198 _]
      tunnel: w180 -> [w197 _]
      tunnel: w182 -> [w196 _]
      tunnel: w181 -> [w195 _]
      tunnel: w174 -> [w194 _]
      frame False {
        n86 = flat-sequence {
          tunnel: w201 -> [w242]
          tunnel: w200 -> [w213]
          tunnel: w199 -> [w233]
          tunnel: w198 -> [w232]
          tunnel: [w210] -> w205
          tunnel: [w218] -> w204
          tunnel: [w233] -> w203
          tunnel: [w232] -> w202
          tunnel: w197 -> [w216]
          tunnel: w196 -> [w224]
          tunnel: w195 -> [w223]
          tunnel: w194 -> [w208]
          tunnel: w205 -> [w248]
          tunnel: w204 -> [w246]
          tunnel: w203 -> [w247]
          tunnel: w202 -> [w249]
          frame #0 {
            n87 = in-place {
              in-place-border: [w244] -> w207
              n88 = in-place-dvr #11(w208) -> (w244:T50)  [unwired: 1 out]
              n89 = in-place-dvr #11() -> ()  [unwired: 1 in, 2 out]
            }
            n90 = local read "Com UDP"() -> (w222:T13)
            n91 = Build Array("Team", "Side") -> (w228:u16[])
            n92 = Build Array("Id camera\nsup esq", "Id camera\ninf esq", "Id camera\ninf dir", "Id camera\nsup dir") -> (w229:dbl[])
            n93 = call "receiveDecodeAndDoKalman.vi"("Vision in"=w224, "NewCameras"=w216, "Field Size"=w223, "Estimador"="Estimador", "cameras array"=w229, "team/side"=w228, "timeToValidateBall"="timeToValidateBall", "Com UDP"=w222, "BallOut"="BallOut", "Life Time"="Life Time", "max ball vel"="ball velocity máx") -> ("Vision out"=w226:refnum<class "Vision.lvclass">, "Frame and Field Size out"=w218:T45, "error out"=w227:errorcluster)  [unwired: 6 in]
            n94 = in-place {
              in-place-border: [w245] -> w243
              n95 = in-place-dvr #12(w242) -> (w245:T32)  [unwired: 1 out]
              n96 = in-place-dvr #12() -> ()  [unwired: 1 in, 2 out]
            }
            n97 = local read "Debug"() -> (w219:bool)
            n98 = local read "Debug Ball"() -> (w220:bool)
            n99 = call "teamAndSide.vi"("Vision in"=w226, "Goalie"="Goalie", "Field State Input"=w218, "Estimador"="Estimador", "Game Status"=w243, "error in (no error)"=w227, "team/side"=w228, "Debug Ball"=w220, "Debug"=w219) -> ("IA State"=w212:T53, "error out"=w211:errorcluster)  [unwired: 4 in, 1 out]
            n100 = local read "touch"() -> (w221:bool)
            n101 = call "oldVisionToGame.vi"("SSL_BallModelStraightTwoPhase"=w207, "Defense stretch"="Defense\n stretch", "Team/ Side"=w228, "Defense width"="Defense\n width", "error in (no error)"=w211, "touch"=w221, "IA State"=w212, "Game in"=w213) -> ("topSpeed"=→"topSpeed":dbl, "Game out"=w210:refnum<class "Game.lvclass">)  [unwired: 1 in, 1 out]
            n102 = call "FPS Counter.vi"() -> ("FPS"=→"FPS vision":dbl)  [unwired: 11 in]
            "Team out" <- "Team"
            "Side out" <- "Side"
          }
          frame #1 {
            n103 = in-place {
              in-place-border: w248 -> [w252]
              n104 = in-place-dvr #13(w249) -> (w253:refnum<class "Game.lvclass">)  [unwired: 1 out]
              n105 = call "BundleAll.vi"("Game in\nvision atualized"=w252, "Game in from reference"=w253) -> ("Game out"=w251:refnum<class "Game.lvclass">)  [unwired: 8 in, 1 out]
              n106 = in-place-dvr #13(w251) -> ()  [unwired: 2 out]
            }
            n107 = in-place {
              in-place-border: w246 -> [w250]
              n108 = in-place-dvr #14(w247) -> ()  [unwired: 2 out]
              n109 = in-place-dvr #14(w250) -> ()  [unwired: 2 out]
            }
          }
        }
      }
      frame True {
      }
    }
    n110 = call "FPS Counter.vi"() -> ("FPS"=→"FPS getCam":dbl)  [unwired: 11 in]
    n111 = Divide(x=1000.0, y=80.0) -> (x/y=w176:dbl)
    n112 = Wait (ms)(milliseconds to wait=w176) -> ()  [unwired: 1 out]
  }
  n113 = while {
    shift-right: [w263] -> _
    shift-left: 0.5 ("New Scale") -> [w270]
    shift-right: [w265] -> _
    shift-left: TRUE ("AutoScale Out") -> [w271]
    tunnel: w19 -> [w269]
    tunnel: w8 -> [w268]
    tunnel: w20 -> [w267]
    stop <- FALSE stop-if-true
    # "Wait necessario\npara 25 FPS"
    # "Draw Field"
    n114 = local read "grSimTest"() -> (w254:bool)
    n115 = call "FPS Counter.vi"() -> ("FPS"=→"FPS Draw Field":dbl)  [unwired: 11 in]
    n116 = Divide(x=1000.0, y=30.0) -> (x/y=w257:dbl)
    n117 = Wait (ms)(milliseconds to wait=w257) -> ()  [unwired: 1 out]
    n118 = feedback #15(0.5 ("New Scale")) -> (w262:dbl)
    n119 = feedback #16(TRUE ("AutoScale Out")) -> (w264:bool)
    n120 = case shown="True" "Draw Field" {
      tunnel: [w272 w284] -> w263
      tunnel: [w273 w283] -> w265
      tunnel: w271 -> [_ w282]
      tunnel: w270 -> [_ w281]
      tunnel: w269 -> [_ w280]
      tunnel: w268 -> [_ w279]
      tunnel: w267 -> [_ w278]
      tunnel: w264 -> [w273 _]
      tunnel: w262 -> [w272 _]
      tunnel: w254 -> [_ w274]
      frame False {
      }
      frame True {
        n121 = flat-sequence {
          tunnel: w282 -> [w294]
          tunnel: w281 -> [w293]
          tunnel: w280 -> [w290]
          tunnel: w279 -> [w289]
          tunnel: w278 -> [w288]
          tunnel: [w296] -> w277
          tunnel: [w295] -> w276
          tunnel: [w286] -> w275
          tunnel: w274 -> [w285]
          tunnel: [w308] -> w283
          tunnel: [w309] -> w284
          tunnel: w277 -> [w309]
          tunnel: w276 -> [w308]
          tunnel: w275 -> [w307]
          frame #0 {
            n122 = disable-structure shown="Enabled" {
              disable-tunnel: [w298 1.0 ("Zoom")] -> w292
              frame Enabled {
                n123 = event shown="[0] \"2D Picture\": Mouse Wheel" {
                  selector: _ -> [_ _]
                  dyn-events: _ -> [_ _]
                  timeout: 0 -> [_ _]
                  tunnel: [w299 1.0] -> w298
                  event "2D Picture": Mouse Wheel {
                    n124 = event-data() -> ("Delta"=w303:i32)  [unwired: 1 in]
                    n125 = Greater Than 0?(x=w303) -> (x > 0?=w302:bool)
                    n126 = Select(t=1.2, s=w302, f=0.8) -> (s? t:f=w299:dbl)
                  }
                  event Timeout {
                    n127 = event-data() -> ()  [unwired: 1 in, 3 out]
                  }
                }
              }
              frame Disabled {
              }
            }
            n128 = in-place {
              in-place-border: [w306] -> w287
              n129 = in-place-dvr #17(w288) -> (w306:T45)  [unwired: 1 out]
              n130 = in-place-dvr #17() -> ()  [unwired: 1 in, 2 out]
            }
            n131 = call "drawField.vi"("Vision in"=w290, "AutoScale"=w294, "Game reference"=w289, "Field State Input"=w287, "grsimtest"=w285, "Scale mm/pixel"=w293, "Draw Targets?"="Draw Targets?", "Zoom"=w292) -> ("AutoScale Out"=w295:bool, "2D Picture"=w286:picture, "Scale Out"=w296:dbl)  [unwired: 3 in, 2 out]
          }
          frame #1 {
            n132 = property on="2D Picture" class="Pict"("Value"=w307) -> ()  [unwired: 2 in, 2 out]
            "2D Picture" <- w307
          }
        }
      }
    }
    n133 = feedback-in #15(w263) -> ()
    n134 = feedback-in #16(w265) -> ()
  }
  n135 = while {
    tunnel: w8 -> [w315]
    stop <- FALSE stop-if-true
    # "grSimTest"
    n136 = case shown="True" "grSimTest" {
      tunnel: w315 -> [_ w324]
      tunnel: [FALSE ("replaceRobots") w320] -> w311
      tunnel: [FALSE ("replaceBall") w319] -> w310
      frame False {
        n137 = Wait (ms)(milliseconds to wait=u32 1000) -> ()  [unwired: 1 out]
      }
      frame True {
        n138 = flat-sequence {
          tunnel: w324 -> [w338]
          tunnel: [w338] -> w326
          tunnel: [w337] -> w325
          tunnel: [w331] -> w320
          tunnel: [w329] -> w319
          tunnel: w326 -> [w342]
          tunnel: w325 -> [w341]
          frame #0 {
            n139 = in-place {
              in-place-border: [w340] -> w339
              n140 = in-place-dvr #18(w338) -> (w340:refnum<class "Game.lvclass">)  [unwired: 1 out]
              n141 = in-place-dvr #18() -> ()  [unwired: 1 in, 2 out]
            }
            n142 = call "grSimTest.vi"("Game in"=w339, "RobotModelFolder"="RobotModelFolder\nFrom RobotModel", "Reaplacement Tests"="Reaplacement Tests", "accel"="accel", "Test"="Test") -> ("velocityPlanningState"=→"velocityPlanningState":T39, "State"=→"RobotModelState":T33, "TestTeam"=w337:refnum<class "Ally.lvclass">, "kickForceTestState"=→"kickForceTestState":T41, "replaceRobots"=w331:bool, "grSIM replacement"=→"grSIM replacement":T6, "replaceBall"=w329:bool)  [unwired: 2 in, 2 out]
          }
          frame #1 {
            n143 = in-place {
              in-place-border: w341 -> [w344]
              n144 = in-place-dvr #19(w342) -> (w345:refnum<class "Game.lvclass">)  [unwired: 1 out]
              n145 = property class="Game"(reference=w345, "TestTeam"=w344) -> (reference out=w343:refnum<class "Game.lvclass">)  [unwired: 1 in, 1 out]
              n146 = in-place-dvr #19(w343) -> ()  [unwired: 2 out]
            }
          }
        }
        n147 = Divide(x=1000.0, y=100.0) -> (x/y=w321:dbl)
        n148 = Wait (ms)(milliseconds to wait=w321) -> ()  [unwired: 1 out]
      }
    }
    "replaceRobots" <- w311
    "replaceBall" <- w310
    n149 = call "FPS Counter.vi"() -> ("FPS"=→"FPS grSimTest":dbl)  [unwired: 11 in]
  }
  n150 = disable-structure shown="Enabled" {
    disable-tunnel: w8 -> [w346 _]
    frame Enabled {
      n151 = while {
        tunnel: w346 -> [w350]
        stop <- FALSE stop-if-true
        # "Draw Graphs"
        n152 = case shown="True" "Draw Graphs" {
          tunnel: w350 -> [_ w363]
          frame False {
          }
          frame True {
            n153 = disable-structure shown="Enabled" {
              frame Disabled {
                n154 = local read "FPS vision"() -> (w376:dbl)
                n155 = Bundle("FPS vision"=w376) -> (w375:cluster{"FPS vision":dbl})  [unwired: 1 in]
                n156 = local read "FPS Navigation"() -> (w373:dbl)
                n157 = local read "FPS Offensive"() -> (w374:dbl)
                n158 = local read "FPS Com"() -> (w372:dbl)
                n159 = Bundle("FPS Navigation"=w373) -> ()  [unwired: 1 in, 1 out]
                n160 = Bundle("FPS Com"=w372) -> ()  [unwired: 1 in, 1 out]
                n161 = Bundle("FPS Offensive"=w374) -> ()  [unwired: 1 in, 1 out]
              }
              frame Enabled {
              }
            }
            n162 = in-place {
              in-place-border: [w377] -> w359
              in-place-border: [w377] -> w353
              n163 = in-place-dvr #20(w363) -> (w377:refnum<class "Game.lvclass">)  [unwired: 1 out]
              n164 = in-place-dvr #20() -> ()  [unwired: 1 in, 2 out]
            }
            n165 = call-dynamic "PlotGraphs.vi"("Game in"=w359, "id 1"="id 1", "id 2"="id 2", "id 3"="id 3") -> ("Ball_vel"=w354:cluster{"Modulo":dbl}, "Ball_z"=w355:cluster{dbl}, "Robot 1"=w358:cluster{"Modulo":dbl, "Modulo":dbl}, "Robot 2"=w357:cluster{"Modulo":dbl, "Modulo":dbl}, "Robot 3"=w356:cluster{"Modulo":dbl, "Modulo":dbl})  [unwired: 4 in, 3 out]
            n166 = disable-structure shown="Enabled" {
              disable-tunnel: w358 -> [w371 _]
              disable-tunnel: w357 -> [w370 _]
              disable-tunnel: w356 -> [w369 _]
              disable-tunnel: w355 -> [w368 _]
              disable-tunnel: w354 -> [w367 _]
              disable-tunnel: w353 -> [w366 _]
              disable-tunnel: "pass?" -> [w364 _]
              frame Enabled {
                n167 = call "BuildGraph.vi"("pass?"=w364, "reference"=w366) -> ("Intensity Graph"=→"Intensity Graph":dbl[][])  [unwired: 7 in, 2 out]
                "Robot" <- w370
                "Robot 2" <- w371
                "Robot" <- w369
                "Ball_z" <- w368
                "Ball_vel" <- w367
              }
              frame Disabled {
              }
            }
          }
        }
        n168 = Wait (ms)(milliseconds to wait=u32 45) -> ()  [unwired: 1 out]
        n169 = call "FPS Counter.vi"() -> ("FPS"=→"FPS Graph":dbl)  [unwired: 11 in]
      }
    }
    frame Disabled {
    }
  }
  n170 = while {
    tunnel: w8 -> [w402]
    stop <- FALSE stop-if-true
    # "Set Parameters"
    n171 = flat-sequence {
      tunnel: w402 -> [w433]
      tunnel: [w433] -> w398
      tunnel: ["Offensive ids"] -> w397
      tunnel: ["Defensive ids"] -> w396
      tunnel: ["zigzag Points"] -> w395
      tunnel: ["TestMode IDS"] -> w394
      tunnel: ["TestMode"] -> w393
      tunnel: ["Tests"] -> w392
      tunnel: ["Test"] -> w391
      tunnel: [w424] -> w390
      tunnel: ["AttakingOurselves"] -> w389
      tunnel: ["Debug"] -> w388
      tunnel: ["ChipKick activated"] -> w387
      tunnel: ["PID gains Vel D"] -> w386
      tunnel: ["PID gains Angle"] -> w385
      tunnel: ["PID gains Lateral"] -> w384
      tunnel: ["Project"] -> w383
      tunnel: ["PID gains Angle To Turn"] -> w381
      tunnel: [w423] -> w380
      tunnel: [w427] -> w379
      tunnel: ["PID gains Radius To Turn"] -> w378
      tunnel: w398 -> [w462]
      tunnel: w397 -> [w464]
      tunnel: w396 -> [w463]
      tunnel: w395 -> [w461]
      tunnel: w394 -> [w460]
      tunnel: w393 -> [w459]
      tunnel: w392 -> [w458]
      tunnel: w391 -> [w457]
      tunnel: w390 -> [w456]
      tunnel: w389 -> [w455]
      tunnel: w388 -> [w454]
      tunnel: w387 -> [w453]
      tunnel: w386 -> [w452]
      tunnel: w385 -> [w451]
      tunnel: w384 -> [w450]
      tunnel: w383 -> [w449]
      tunnel: w381 -> [w448]
      tunnel: w380 -> [w447]
      tunnel: w379 -> [w446]
      tunnel: w378 -> [w445]
      frame #0 {
        n172 = local read "Com UDP"() -> (w419:T13)
        n173 = local read "RefBox UDP RX"() -> (w420:T12)
        n174 = local read "Command"() -> (w418:string)
        n175 = local read "Goalie"() -> (w417:string)
        n176 = local read "SSL UDP RX"() -> (w421:T12)
        n177 = local read "Side"() -> (w416:enum16{"Esquerdo", "Direito"})
        n178 = local read "Team"() -> (w415:enum16{"Azul", "Amarelo"})
        n179 = Bundle By Name(cluster=T68 {"SSL UDP RX"={"Local IP:"="", "Server IP:"="224.5.23.2", "Port"="10020"}, "RefBox UDP RX"={"Local IP:"="", "Server IP:"="224.5.23.1", "Port"="10003"}, "Com UDP"={"UDP GrSim TX"=TRUE, "Address:"="172.29.47.23", "Port:"=10301}, "Command"="Force Start", "Goalie"="0", "Side"=enum."Esquerdo", "Team"=enum."Azul"} ("MainGameConfigs"), "SSL UDP RX"=w421, "RefBox UDP RX"=w420, "Com UDP"=w419, "Command"=w418, "Goalie"=w417, "Side"=w416, "Team"=w415) -> (w414:T68)
        n180 = call "chooseParametersFromFiles.vi"("AI Parameters"="AI Parameters", "NewParameters"="NewParameters", "MainGameConfigs"=w414, "ParametersFromFile"="ParametersFromFile") -> ("AI Parameters out"=w424:T20, "NewParameters out"=w423:T26, "MainGameConfigs out"=w413:T68)  [unwired: 11 in, 2 out]
        n181 = Unbundle By Name(w413) -> ("SSL UDP RX"=w412:T12, "RefBox UDP RX"=w411:T12, "Com UDP"=w410:T13, "Command"=w409:string, "Goalie"=w408:string, "Side"=w407:enum16{"Esquerdo", "Direito"}, "Team"=w406:enum16{"Azul", "Amarelo"})
        n182 = local write "SSL UDP RX"(w412) -> ()
        n183 = local write "RefBox UDP RX"(w411) -> ()
        n184 = local write "Command"(w409) -> ()
        n185 = local write "Goalie"(w408) -> ()
        n186 = local write "Com UDP"(w410) -> ()
        n187 = local write "Side"(w407) -> ()
        n188 = local write "Team"(w406) -> ()
        n189 = Unbundle By Name(w424) -> ("DefenseAvoidArea"=→"DefenseAvoidArea":bool)
        n190 = local read "Envirnoment"() -> (w427:T17)
      }
      frame #1 {
        n191 = in-place {
          in-place-border: w464 -> [w485]
          in-place-border: w463 -> [w484]
          in-place-border: w461 -> [w472]
          in-place-border: w460 -> [w482]
          in-place-border: w459 -> [w481]
          in-place-border: w458 -> [w480]
          in-place-border: w457 -> [w479]
          in-place-border: w456 -> [w478]
          in-place-border: w455 -> [w477]
          in-place-border: w454 -> [w475]
          in-place-border: w453 -> [w476]
          in-place-border: w452 -> [w474]
          in-place-border: w451 -> [w473]
          in-place-border: w450 -> [w470]
          in-place-border: w449 -> [w471]
          in-place-border: w448 -> [w468]
          in-place-border: w447 -> [w467]
          in-place-border: w446 -> [w466]
          in-place-border: w445 -> [w465]
          n192 = in-place-dvr #21(w462) -> (w486:refnum<class "Game.lvclass">)  [unwired: 1 out]
          n193 = call "setParameters.vi"("Game in"=w486, "TestMode"=w481, "PID gains Lateral"=w470, "Tests"=w480, "PID gains Angle"=w473, "zigzag Points"=w472, "AI Parameters"=w478, "PID gains Angle To Turn"=w468, "Project"=w471, "AttakingOurselves"=w477, "Defensive ids"=w484, "ChipKick activated"=w476, "TestMode IDS"=w482, "Debug"=w475, "Offensive ids"=w485, "PID gains Vel D"=w474, "Test"=w479, "NewParameters"=w467, "PID gains Radius To Turn"=w465, "Enviroment"=w466) -> ("Game out"=w483:refnum<class "Game.lvclass">, "error out"=→"error out":errorcluster)  [unwired: 6 in]
          n194 = in-place-dvr #21(w483) -> ()  [unwired: 2 out]
        }
      }
    }
    n195 = call "FPS Counter.vi"() -> ("FPS"=→"FPS SetParameters":dbl)  [unwired: 11 in]
    n196 = Divide(x=1000.0, y=5.0) -> (x/y=w399:dbl)
    n197 = Wait (ms)(milliseconds to wait=w399) -> ()  [unwired: 1 out]
  }
  n198 = while {
    tunnel: w8 -> [w496]
    stop <- FALSE stop-if-true
    # "Event Generator"
    n199 = local read "FPS vision"() -> (w489:dbl)
    n200 = flat-sequence {
      tunnel: w496 -> [w503]
      tunnel: [w500] -> w495
      tunnel: [w499] -> w494
      tunnel: w495 -> [w506]
      tunnel: w494 -> [w505]
      frame #0 {
        n201 = in-place {
          in-place-border: [w504] -> w502
          n202 = in-place-dvr #22(w503) -> (w504:refnum<class "Game.lvclass">)  [unwired: 1 out]
          n203 = in-place-dvr #22() -> (w500:refnum<data-value>)  [unwired: 1 in, 1 out]
        }
        n204 = call-dynamic "Generate_events.vi"("Game in"=w502, "Events in"=refnum<class "Events.lvclass"> refnum) -> ("kick"=→"kick":bool, "touch"=→"touch":bool, "Events out"=w499:refnum<class "Events.lvclass">)  [unwired: 6 in, 1 out]
      }
      frame #1 {
        n205 = in-place {
          in-place-border: w505 -> [w508]
          n206 = in-place-dvr #23(w506) -> (w509:refnum<class "Game.lvclass">)  [unwired: 1 out]
          n207 = property class="Game"(reference=w509, "EventsRef"=w508) -> (reference out=w507:refnum<class "Game.lvclass">)  [unwired: 1 in, 1 out]
          n208 = in-place-dvr #23(w507) -> ()  [unwired: 2 out]
        }
      }
    }
    n209 = Subtract(x=w489, y=2.0) -> (x-y=w487:dbl)
    n210 = call "FPS Counter.vi"() -> ("FPS"=→"FPS Events":dbl)  [unwired: 11 in]
    n211 = Divide(x=1000.0, y=w487) -> (x/y=w490:dbl)
    n212 = Wait (ms)(milliseconds to wait=w490) -> ()  [unwired: 1 out]
  }
  n213 = while {
    tunnel: w8 -> [w517]
    stop <- FALSE stop-if-true
    # "Offensive"
    n214 = flat-sequence {
      tunnel: w517 -> [w529]
      tunnel: [w522] -> w516
      tunnel: [w524] -> w515
      tunnel: [w523] -> w514
      tunnel: w516 -> [w533]
      tunnel: w515 -> [w532]
      tunnel: w514 -> [w531]
      frame #0 {
        n215 = in-place {
          in-place-border: [w530] -> w519
          n216 = in-place-dvr #24(w529) -> (w530:refnum<class "Game.lvclass">)  [unwired: 1 out]
          n217 = in-place-dvr #24() -> (w523:refnum<data-value>)  [unwired: 1 in, 1 out]
        }
        n218 = call "chooseOffensivePlay.vi"("Game"=w519) -> ("error out"=w527:errorcluster, "Game out"=w526:refnum<class "Game.lvclass">, "Plays"=→"LastOffensivePlays":T2[])  [unwired: 5 in, 3 out]
        n219 = call-dynamic "pickOffensiveRobots.vi"("error in (no error)"=w527, "Game in"=w526) -> ("error out"=w528:errorcluster, "Game out"=w525:refnum<class "Game.lvclass">)  [unwired: 8 in]
        n220 = call "executeOffensivePlay.vi"("error in (no error)"=w528, "Game in"=w525) -> ("Game out"=w520:refnum<class "Game.lvclass">)  [unwired: 8 in, 1 out]
        n221 = property class="Game"(reference=w520) -> ("OffensiveTeam"=w522:refnum<class "Ally.lvclass">, "Playbook"=w524:refnum<class "Playbook.lvclass">)  [unwired: 1 in, 2 out]
      }
      frame #1 {
        n222 = in-place {
          in-place-border: w533 -> [w537]
          in-place-border: w532 -> [w536]
          n223 = in-place-dvr #25(w531) -> (w534:refnum<class "Game.lvclass">)  [unwired: 1 out]
          n224 = property class="Game"(reference=w534, "OffensiveTeam"=w537, "Playbook"=w536) -> (reference out=w535:refnum<class "Game.lvclass">)  [unwired: 1 in, 1 out]
          n225 = in-place-dvr #25(w535) -> ()  [unwired: 2 out]
        }
      }
    }
    n226 = Divide(x=1000.0, y=80.0) -> (x/y=w511:dbl)
    n227 = Wait (ms)(milliseconds to wait=w511) -> ()  [unwired: 1 out]
    n228 = call "FPS Counter.vi"() -> ("FPS"=→"FPS Offensive":dbl)  [unwired: 11 in]
  }
  n229 = while {
    tunnel: w8 -> [w545]
    stop <- FALSE stop-if-true
    # "Keeper"
    n230 = flat-sequence {
      tunnel: w545 -> [w553]
      tunnel: [w551] -> w544
      tunnel: [w550] -> w543
      tunnel: [w549] -> w542
      tunnel: [w562] -> _
      tunnel: w544 -> [w562]
      tunnel: w543 -> [w561]
      tunnel: w542 -> [w560]
      frame #0 {
        n231 = in-place {
          in-place-border: [w559] -> w547
          n232 = in-place-dvr #26(w553) -> (w559:refnum<class "Game.lvclass">)  [unwired: 1 out]
          n233 = in-place-dvr #26() -> (w551:refnum<data-value>)  [unwired: 1 in, 1 out]
        }
        n234 = call "chooseKeeperPlay.vi"("Game in"=w547) -> ("error out"=w557:errorcluster, "Game out"=w552:refnum<class "Game.lvclass">)  [unwired: 9 in]
        n235 = call "pickKeeperRobots.vi"("error in (no error)"=w557, "Game in"=w552) -> ("error out"=w558:errorcluster, "Game out"=w555:refnum<class "Game.lvclass">)  [unwired: 8 in]
        n236 = call "executeKeeperPlay.vi"("error in (no error)"=w558, "Game in"=w555) -> ("error out"=w556:errorcluster, "Game out"=w554:refnum<class "Game.lvclass">)  [unwired: 8 in]
        n237 = call-dynamic "pathPlanningKeeper.vi"("error in (no error)"=w556, "Game in"=w554) -> ("Game out"=w548:refnum<class "Game.lvclass">)  [unwired: 8 in, 1 out]
        n238 = property class="Game"(reference=w548) -> ("KeeperTeam"=w550:refnum<class "Ally.lvclass">, "Playbook"=w549:refnum<class "Playbook.lvclass">)  [unwired: 1 in, 2 out]
      }
      frame #1 {
        n239 = in-place {
          in-place-border: w561 -> [w564]
          in-place-border: w560 -> [w565]
          n240 = in-place-dvr #27(w562) -> (w563:refnum<class "Game.lvclass">)  [unwired: 1 out]
          n241 = property class="Game"(reference=w563, "KeeperTeam"=w564, "Playbook"=w565) -> (reference out=w566:refnum<class "Game.lvclass">)  [unwired: 1 in, 1 out]
          n242 = in-place-dvr #27(w566) -> ()  [unwired: 2 out]
        }
      }
    }
    n243 = call "FPS Counter.vi"() -> ("FPS"=→"FPS Keeper":dbl)  [unwired: 11 in]
    n244 = Divide(x=1000.0, y=80.0) -> (x/y=w540:dbl)
    n245 = Wait (ms)(milliseconds to wait=w540) -> ()  [unwired: 1 out]
  }
  n246 = while {
    tunnel: w8 -> [w574]
    stop <- FALSE stop-if-true
    # "Defensive"
    n247 = flat-sequence {
      tunnel: w574 -> [w587]
      tunnel: [w580] -> w573
      tunnel: [w579] -> w572
      tunnel: [w578] -> w571
      tunnel: w573 -> [w590]
      tunnel: w572 -> [w589]
      tunnel: w571 -> [w591]
      frame #0 {
        n248 = in-place {
          in-place-border: [w588] -> w576
          n249 = in-place-dvr #28(w587) -> (w588:refnum<class "Game.lvclass">)  [unwired: 1 out]
          n250 = in-place-dvr #28() -> (w578:refnum<data-value>)  [unwired: 1 in, 1 out]
        }
        n251 = call-dynamic "chooseDefensivePlay.vi"("Game in"=w576) -> ("error out"=w585:errorcluster, "Game out"=w586:refnum<class "Game.lvclass">)  [unwired: 9 in]
        n252 = call-dynamic "pickDefensiveRobots.vi"("error in (no error)"=w585, "Game in"=w586) -> ("error out"=w583:errorcluster, "Game out"=w584:refnum<class "Game.lvclass">)  [unwired: 8 in]
        n253 = call-dynamic "executeDefensivePlay.vi"("error in (no error)"=w583, "Game in"=w584) -> ("error out"=w582:errorcluster, "Game out"=w581:refnum<class "Game.lvclass">)  [unwired: 8 in]
        n254 = call-dynamic "pathPlanningDefensive.vi"("error in (no error)"=w582, "Game in"=w581) -> ("Game out"=w577:refnum<class "Game.lvclass">)  [unwired: 8 in, 1 out]
        n255 = property class="Game"(reference=w577) -> ("DefensiveTeam"=w580:refnum<class "Ally.lvclass">, "Playbook"=w579:refnum<class "Playbook.lvclass">)  [unwired: 1 in, 2 out]
      }
      frame #1 {
        n256 = in-place {
          in-place-border: w590 -> [w593]
          in-place-border: w589 -> [w594]
          n257 = in-place-dvr #29(w591) -> (w592:refnum<class "Game.lvclass">)  [unwired: 1 out]
          n258 = property class="Game"(reference=w592, "DefensiveTeam"=w593, "Playbook"=w594) -> (reference out=w595:refnum<class "Game.lvclass">)  [unwired: 1 in, 1 out]
          n259 = in-place-dvr #29(w595) -> ()  [unwired: 2 out]
        }
      }
    }
    n260 = Divide(x=1000.0, y=80.0) -> (x/y=w569:dbl)
    n261 = Wait (ms)(milliseconds to wait=w569) -> ()  [unwired: 1 out]
    n262 = call "FPS Counter.vi"() -> ("FPS"=→"FPS Defensive":dbl)  [unwired: 11 in]
  }
  n263 = while {
    tunnel: w8 -> [w598]
    stop <- FALSE stop-if-true
    # "RRTOffensive"
    n264 = local read "DefenseAvoidArea"() -> (w596:bool)
    n265 = Divide(x=1000.0, y=80.0) -> (x/y=w602:dbl)
    n266 = Wait (ms)(milliseconds to wait=w602) -> ()  [unwired: 1 out]
    n267 = call "rrtOffensiveWhile.vi"("AttackerAvoidArea"="AttackerAvoidArea", "Line?"="Line?", "Volta ao redor\nda área?"=w596, "GameReference in"=w598) -> ()  [unwired: 7 in, 1 out]
    n268 = call "FPS Counter.vi"() -> ("FPS"=→"FPS RRTOffensive":dbl)  [unwired: 11 in]
  }
  n269 = while {
    tunnel: w8 -> [w608]
    stop <- FALSE stop-if-true
    # "Navigation"
    n270 = flat-sequence {
      tunnel: [w627] -> w612
      tunnel: w608 -> [w626]
      tunnel: [w617] -> w607
      tunnel: [w620] -> w606
      tunnel: [w654] -> _
      tunnel: w612 -> [w654]
      tunnel: w607 -> [w652]
      tunnel: w606 -> [w653]
      frame #0 {
        # "GAMBIARRA"
        n271 = in-place {
          in-place-border: [w649] -> w628
          n272 = in-place-dvr #30(w626) -> (w649:refnum<class "Game.lvclass">)  [unwired: 1 out]
          n273 = in-place-dvr #30() -> (w627:refnum<data-value>)  [unwired: 1 in, 1 out]
        }
        n274 = disable-structure shown="Enabled" {
          disable-tunnel: w628 -> [w648 _]
          disable-tunnel: [w646 _] -> w624
          frame Disabled {
            n275 = call "NavigationDefensive.vi"("Game in"=w648) -> ("Game out"=w647:refnum<class "Game.lvclass">)  [unwired: 9 in, 1 out]
            n276 = property class="Game"(reference=w647) -> ("DefensiveTeam"=w645:refnum<class "Ally.lvclass">)  [unwired: 1 in, 2 out]
            n277 = property class="Ally"(reference=w645) -> ("RobotRef"=w646:refnum<class "Robot.lvclass">[])  [unwired: 1 in, 2 out]
          }
          frame Enabled {
          }
        }
        n278 = call "NavigationOffensive.vi"("Game in"=w628) -> ("NaN?"=→"NaN?":bool, "Game out"=w619:refnum<class "Game.lvclass">)  [unwired: 7 in, 2 out]
        n279 = call "NavigationKeeper.vi"("Game in"=w628) -> ("Game out"=w621:refnum<class "Game.lvclass">)  [unwired: 9 in, 1 out]
        n280 = property class="Game"(reference=w619) -> ("OffensiveTeam"=w622:refnum<class "Ally.lvclass">)  [unwired: 1 in, 2 out]
        n281 = property class="Game"(reference=w621) -> ("AllyRef"=w620:refnum<class "Ally.lvclass">)  [unwired: 1 in, 2 out]
        n282 = property class="Game"(reference=w621) -> ("KeeperTeam"=w616:refnum<class "Ally.lvclass">, "KeeperTeam"=w623:refnum<class "Ally.lvclass">)  [unwired: 1 in, 2 out]
        n283 = property class="Ally"(reference=w616) -> ("KeeperPlay"=w615:T3)  [unwired: 1 in, 2 out]
        n284 = property class="Ally"(reference=w623) -> ("RobotRef"=w625:refnum<class "Robot.lvclass">[])  [unwired: 1 in, 2 out]
        n285 = property class="Ally"(reference=w622) -> ("RobotRef"=w614:refnum<class "Robot.lvclass">[])  [unwired: 1 in, 2 out]
        n286 = case shown="\"ZigZag\", Default" w615 {
          tunnel: w625 -> [w634 w644]
          tunnel: w614 -> [w631 _]
          tunnel: w624 -> [w630 _]
          tunnel: [w629 w644] -> w617
          frame "ZigZag", Default {
            n287 = for {
              tunnel: w634 -> [w643] mode=indexing
              shift-right: [w641] -> w632
              shift-left: refnum<class "Robot.lvclass">[] [] -> [w642]
              n288 = Insert Into Array(array=w642, new element=w643) -> (w641:refnum<class "Robot.lvclass">[])  [unwired: 1 in]
            }
            n289 = for {
              tunnel: w631 -> [w640] mode=indexing
              shift-right: [w638] -> w629
              shift-left: w632 -> [w639]
              n290 = Insert Into Array(array=w639, new element=w640) -> (w638:refnum<class "Robot.lvclass">[])  [unwired: 1 in]
            }
            n291 = for {
              tunnel: w630 -> [w637] mode=indexing
              shift-right: [w635] -> _
              shift-left: w629 -> [w636]
              n292 = Insert Into Array(array=w636, new element=w637) -> (w635:refnum<class "Robot.lvclass">[])  [unwired: 1 in]
            }
          }
          frame "BallPlacementAlly" {
          }
        }
      }
      frame #1 {
        # "192.168.2.61"
        n293 = in-place {
          in-place-border: w652 -> [w658]
          in-place-border: w653 -> [w657]
          n294 = in-place-dvr #31(w654) -> (w656:refnum<class "Game.lvclass">)  [unwired: 1 out]
          n295 = property class="Ally"(reference=w657, "RobotRef"=w658) -> (reference out=w659:refnum<class "Ally.lvclass">)  [unwired: 1 in, 1 out]
          n296 = property class="Game"(reference=w656, "NavigationTeam"=w659) -> (reference out=w655:refnum<class "Game.lvclass">)  [unwired: 1 in, 1 out]
          n297 = in-place-dvr #31(w655) -> ()  [unwired: 2 out]
        }
        n298 = call "FindRobotByID.vi"("id"=1, "RobotRef"=w652) -> ("Robot"=w650:refnum<class "Robot.lvclass">)  [unwired: 6 in, 3 out]
        n299 = property class="Robot" props=["debug_v_norm", "debug_v_tang"](reference=w650) -> ()  [unwired: 1 in, 4 out]
      }
    }
    n300 = call "FPS Counter.vi"() -> ("FPS"=→"FPS Navigation":dbl)  [unwired: 11 in]
    n301 = Divide(x=1000.0, y=100.0) -> (x/y=w611:dbl)
    n302 = Wait (ms)(milliseconds to wait=w611) -> ()  [unwired: 1 out]
  }
  n303 = disable-structure shown="Disabled" {
    frame Disabled {
      "Exit" <- 0 ("Exit")
      "Log" <- "safe" ("Log")
    }
    frame Enabled {
    }
  }
  n304 = while {
    tunnel: w8 -> [w672]
    stop <- FALSE stop-if-true
    # "ErForceSimulatorReplacement"
    n305 = in-place {
      in-place-border: [w676] -> w662
      n306 = in-place-dvr #32(w672) -> (w676:refnum<class "Game.lvclass">)  [unwired: 1 out]
      n307 = in-place-dvr #32() -> ()  [unwired: 1 in, 2 out]
    }
    n308 = local read "grSIM replacement"() -> (w668:T6)
    n309 = local read "Com UDP"() -> (w669:T13)
    n310 = local read "replaceBall"() -> (w663:bool)
    n311 = local read "Debug Ball"() -> (w667:bool)
    n312 = local read "Debug"() -> (w666:bool)
    n313 = call "FPS Counter.vi"() -> ("FPS"=→"FPS ReplaceErForce":dbl)  [unwired: 11 in]
    n314 = And(x=w667, y=w666) -> (x .and. y?=w665:bool)
    n315 = local read "replaceRobots"() -> (w664:bool)
    n316 = call "communicateReplacementErForceSimulator.vi"("replaceBall"=w663, "degubBall"=w665, "Com UDP"=w669, "grSIM replacement"=w668, "Game"=w662, "replaceRobots"=w664) -> ()  [unwired: 8 in, 2 out]
    n317 = Divide(x=1000.0 ("y"), y=70.0) -> (x/y=w673:dbl)
    n318 = Wait (ms)(milliseconds to wait=w673) -> ()  [unwired: 1 out]
  }
  n319 = global write "commCAS.vi" "CommCAS"(0.0) -> ()
  n320 = New Data Value Reference(data value=T19[] [] ("displayFeedbackRobot 2")) -> (data value reference=w6:refnum<data-value>)  [unwired: 1 in, 1 out]
  n321 = while {
    tunnel: w8 -> [w682]
    tunnel: w6 -> [w678]
    stop <- FALSE stop-if-true
    # "RobotControlResponse"
    n322 = flat-sequence {
      tunnel: [w688] -> w683
      tunnel: w682 -> [w691]
      tunnel: [w693] -> w681
      tunnel: w678 -> [w687]
      tunnel: w683 -> [w720]
      tunnel: w681 -> [w719]
      frame #0 {
        n323 = in-place {
          in-place-border: [w696] -> w694
          n324 = in-place-dvr #33(w691) -> (w696:refnum<class "Game.lvclass">)  [unwired: 1 out]
          n325 = in-place-dvr #33() -> (w693:refnum<data-value>)  [unwired: 1 in, 1 out]
        }
        n326 = local read "Com Serial"() -> (w692:T14)
        n327 = Unbundle By Name(w692) -> ("Serial TX"=w690:bool)
        n328 = case shown="True" w690 {
          tunnel: [w697 w701] -> w689
          tunnel: w694 -> [w700 _]
          tunnel: w692 -> [w699 _]
          frame True {
            n329 = call "receiveSerialFeedback.vi"("robotAngles"="robotAngles", "Com Serial"=w699, "Game"=w700) -> ("RobotsFeedback"=w697:refnum<class "RobotFeedback.lvclass">[])  [unwired: 6 in, 2 out]
          }
          frame False {
            n330 = local read "robotControlResponseConnectionID"() -> (w703:refnum<k16>)
            n331 = UDP Read(connection ID=w703) -> (data out=w706:string, error out=→"error out 2":errorcluster)  [unwired: 3 in, 3 out]
            n332 = String To Byte Array(string=w706) -> (unsigned byte array=w705:u8[])
            n333 = call "sslSimulationProtocolRobotControlResponse.vi"("robotControlArray"=w705) -> ("error out"=→"robotControlResponseErrorOut":errorcluster, "RobotsFeedback"=w702:refnum<class "RobotFeedback.lvclass">[])  [unwired: 9 in]
            n334 = disable-structure shown="Enabled" {
              disable-tunnel: w702 -> [w712 _]
              frame Enabled {
                n335 = for {
                  tunnel: w712 -> [w715] mode=indexing
                  tunnel: [w716] -> w711 mode=indexing
                  n336 = property class="RobotFeedback.lvclass"(reference=w715) -> ("id"=w714:i32, "dribblerContactToBall"=w713:bool)  [unwired: 1 in, 2 out]
                  n337 = Bundle By Name(cluster=cluster{"id":u32, "dribblerContact":bool} {"id"=0, "dribblerContact"=FALSE} ("robotFeedback"), "id"=w714, "dribblerContact"=w713) -> (w716:cluster{"id":u32, "dribblerContact":bool})
                }
                "robotFeedback" <- w711
              }
              frame Disabled {
              }
            }
            n338 = disable-structure shown="Enabled" {
              disable-tunnel: w702 -> [w709 w710]
              disable-tunnel: [w708 w710] -> w701
              frame Disabled {
                n339 = call "simulatorCustomFeedbackControl.vi"("RobotsFeedback"=w709) -> ("feedback_array"=w708:refnum<class "RobotFeedback.lvclass">[])  [unwired: 8 in, 2 out]
              }
              frame Enabled {
              }
            }
          }
        }
        n340 = call "displayFeedback.vi"("feedback_array"=w689) -> ("robotDisplayFeedback"=w686:T19[], "feedback_array out"=w688:refnum<class "RobotFeedback.lvclass">[])  [unwired: 7 in, 2 out]
        n341 = in-place {
          in-place-border: w686 -> [w695]
          n342 = in-place-dvr #34(w687) -> ()  [unwired: 2 out]
          n343 = in-place-dvr #34(w695) -> ()  [unwired: 2 out]
        }
      }
      frame #1 {
        n344 = case shown="False" "Boolean" {
          frame False {
          }
          frame True {
            n345 = global write "commCAS.vi" "CommCAS"(1) -> ()
          }
        }
        n346 = in-place {
          in-place-border: w720 -> [w722]
          n347 = in-place-dvr #35(w719) -> (w724:refnum<class "Game.lvclass">)  [unwired: 1 out]
          n348 = property class="Game"(reference=w724, "RobotsFeedback"=w722) -> (reference out=w723:refnum<class "Game.lvclass">)  [unwired: 1 in, 1 out]
          n349 = in-place-dvr #35(w723) -> ()  [unwired: 2 out]
        }
      }
    }
    n350 = Divide(x=2000.0, y=1000.0) -> (x/y=w677:dbl)
    n351 = Wait (ms)(milliseconds to wait=w677) -> ()  [unwired: 1 out]
    n352 = call "FPS Counter.vi"() -> ("FPS"=→"FPS RobotFeedback":dbl)  [unwired: 11 in]
  }
  n353 = while {
    tunnel: w6 -> [w727]
    stop <- FALSE stop-if-true
    # "Draw Feedback"
    n354 = in-place {
      in-place-border: [w732] -> w726
      n355 = in-place-dvr #36(w727) -> (w732:T19[])  [unwired: 1 out]
      n356 = in-place-dvr #36() -> ()  [unwired: 1 in, 2 out]
    }
    "displayFeedbackRobot" <- w726
    n357 = Divide(x=1000.0, y=10.0) -> (x/y=w731:dbl)
    n358 = Wait (ms)(milliseconds to wait=w731) -> ()  [unwired: 1 out]
    n359 = property on="2D Picture" class="Pict"("ZoomFactor"=sgl 0.2 ("Zoom Factor")) -> ()  [unwired: 2 in, 2 out]
  }
  n360 = while {
    tunnel: w8 -> [w755]
    stop <- FALSE stop-if-true
    # "Communication"
    n361 = local read "ReplayControls"() -> (w734:T29)
    n362 = Divide(x=1000.0 ("y"), y=70.0) -> (x/y=w743:dbl)
    n363 = in-place {
      in-place-border: [w756] -> w747
      n364 = in-place-dvr #37(w755) -> (w756:refnum<class "Game.lvclass">)  [unwired: 1 out]
      n365 = in-place-dvr #37() -> ()  [unwired: 1 in, 2 out]
    }
    n366 = Wait (ms)(milliseconds to wait=w743) -> ()  [unwired: 1 out]
    n367 = local read "grSimTest"() -> (w746:bool)
    n368 = local read "grSIM replacement"() -> (w736:T6)
    n369 = local read "replaceRobots"() -> (w735:bool)
    n370 = local read "Debug"() -> (w740:bool)
    n371 = local read "replaceBall"() -> (w742:bool)
    n372 = local read "FIRASim?"() -> (w748:bool)
    n373 = And(x="Debug Ball", y=w740) -> (x .and. y?=w739:bool)
    n374 = call-dynamic "communicate.vi"("Communication in"="Communication in", "Game"=w747, "ReplayControls"=w734, "Com UDP"="Com UDP", "Com Serial"="Com Serial", "grSimTest"=w746, "Com SOS"="Com SOS", "ABORT"="ABORT!!!!!!!!!", "Enviroment"="Envirnoment", "grSIM replacement"=w736, "FIRASim?"=w748, "ReplaceRobots"=w735, "repalceBall"=w742, "Debug"=w739) -> ("Comm TX FPS"=→"FPS Com":dbl, "connection ID out"=→"robotControlResponseConnectionID":refnum<k16>)  [unwired: 2 in, 2 out]
    "Envirnoment out" <- "Envirnoment"
  }
  n375 = while {
    tunnel: w8 -> [w777]
    stop <- FALSE stop-if-true
    # "Debug"
    n376 = in-place {
      in-place-border: [w793] -> w762
      n377 = in-place-dvr #38(w777) -> (w793:refnum<class "Game.lvclass">)  [unwired: 1 out]
      n378 = in-place-dvr #38() -> ()  [unwired: 1 in, 2 out]
    }
    n379 = call "FPS Counter.vi"() -> ("FPS"=→"FPS Debug":dbl)  [unwired: 11 in]
    n380 = property class="Game"(reference=w762) -> ("Referee"=w768:refnum<class "Referee.lvclass">, "KeeperTeam"=w776:refnum<class "Ally.lvclass">, "OffensiveTeam"=w775:refnum<class "Ally.lvclass">, "DefensiveTeam"=w774:refnum<class "Ally.lvclass">)  [unwired: 1 in, 2 out]
    n381 = Divide(x=1000.0, y=60.0) -> (x/y=w761:dbl)
    n382 = Wait (ms)(milliseconds to wait=w761) -> ()  [unwired: 1 out]
    n383 = property class="Referee"(reference=w768) -> ("command_interpreted"=→"command_interpreted":T5)  [unwired: 1 in, 2 out]
    n384 = property class="Ally"(reference=w774) -> ("RobotRef"=w771:refnum<class "Robot.lvclass">[], "DefensivePlay"=→"DefensivePlay":T4)  [unwired: 1 in, 2 out]
    n385 = property class="Ally"(reference=w775) -> ("RobotRef"=w772:refnum<class "Robot.lvclass">[], "OffensivePlay"=→"OffensivePlay":T2)  [unwired: 1 in, 2 out]
    n386 = property class="Ally"(reference=w776) -> ("RobotRef"=w773:refnum<class "Robot.lvclass">[], "KeeperPlay"=→"KeeperPlay":T3)  [unwired: 1 in, 2 out]
    n387 = for {
      tunnel: w772 -> [w787] mode=indexing
      tunnel: [w784] -> w765 mode=indexing
      n388 = property class="Robot"(reference=w787) -> ("id"=w786:i32, "role"=w785:T30, "tactic"=w783:T31)  [unwired: 1 in, 2 out]
      n389 = Bundle("id"=w786, "role"=w785, "tactic"=w783) -> (w784:cluster{"id":i32, "role":T30, "tactic":T31})  [unwired: 1 in]
    }
    "Offensive Team" <- w765
    n390 = for {
      tunnel: w773 -> [w792] mode=indexing
      tunnel: [w789] -> w766 mode=indexing
      n391 = property class="Robot"(reference=w792) -> ("id"=w791:i32, "role"=w790:T30, "tactic"=w788:T31)  [unwired: 1 in, 2 out]
      n392 = Bundle("id"=w791, "role"=w790, "tactic"=w788) -> (w789:cluster{"id":i32, "role":T30, "tactic":T31})  [unwired: 1 in]
    }
    "Keeper Team" <- w766
    n393 = for {
      tunnel: w771 -> [w782] mode=indexing
      tunnel: [w779] -> w764 mode=indexing
      n394 = property class="Robot"(reference=w782) -> ("id"=w781:i32, "role"=w780:T30, "tactic"=w778:T31)  [unwired: 1 in, 2 out]
      n395 = Bundle("id"=w781, "role"=w780, "tactic"=w778) -> (w779:cluster{"id":i32, "role":T30, "tactic":T31})  [unwired: 1 in]
    }
    "Defensive Team" <- w764
  }
